vi "RIB Req - UDP Init.vi"(0 "Limits File Path":path, 5 "Results File Path":path, 11 "error in":errorcluster) -> (4 "Results Data Array":string[][](array[string]), 15 "error out":errorcluster)   [LabVIEW 2024]
doc: "Template test"
uses:
  <vilib>/addons/_JKI Toolkits/State Machine/_JKI_lib_State_Machine.llb/Select State(s)_err__jki_lib_state_machine.vi
  <vilib>/DAQmx/write.llb/DAQmx Write (Digital 1D Bool 1Chan 1Samp).vi
  <vilib>/addons/_JKI Toolkits/State Machine/_JKI_lib_State_Machine.llb/Select State(s)_bool__jki_lib_state_machine.vi
  <vilib>/DAQmx/read.llb/DAQmx Read (Digital 1D Bool 1Chan 1Samp).vi
  <vilib>/addons/_JKI Toolkits/State Machine/_JKI_lib_State_Machine.llb/Periodic Trigger__ogtk__JKI-SM__jki_lib_state_machine.vi
  <userlib>/_OpenG.lib/file/file.llb/Strip Path Extension - String__ogtk.vi
  <vilib>/Utility/file.llb/Read Delimited Spreadsheet (string).vi
  <vilib>/Utility/file.llb/Write Delimited Spreadsheet (string).vi
  <vilib>/DAQmx/create/channels.llb/DAQmx Create Channel (DO-Digital Output).vi
  <vilib>/DAQmx/miscellaneous.llb/DAQmx Fill In Error Info.vi
  <userlib>/_OpenG.lib/file/file.llb/openg_file.lvlib
  <userlib>/_OpenG.lib/appcontrol/appcontrol.llb/openg_application_control.lvlib
  <userlib>/_OpenG.lib/time/time.llb/openg_time.lvlib
panel:
  in  "Connect":string
  in  "Connect Fail":string
  out "data out":string
  out "Timeout (Read States) 4":dbl(slide) scale=0.0..10.0
  out "Timeout (Read States) 3":dbl(slide) scale=0.0..10.0
  out "Timeout (Read States) 2":dbl(slide) scale=0.0..10.0
  out "Timeout (Read States)":dbl(slide) scale=0.0..15.0
  out "element":string
  out "5A Test":bool
  out "ROV A Enabled":bool
  out "ROV B Enabled":bool
  out "TMS Enabled":bool
  out "Wait for Start":bool
  out "Normal Operation":bool
  in  "Read Normal Operation":string
  in  "Read Wait for Start":string
  in  "Read TMS":string
  in  "Read ROV B":string
  in  "Read ROV A":string
  out "Results Data 10":string[](array[string])
  out "Results Data 9":string[](array[string])
  out "Results Data 8":string[](array[string])
  out "Results Data 7":string[](array[string])
  out "Results Data 6":string[](array[string])
  out "Results Data 5":string[](array[string])
  out "Results Data 4":string[](array[string])
  in  "5A Test":bool
  out "Results Data 3":string[](array[string])
  in  "task out":refnum<k21>
  out "Timeout (5A)":dbl(slide) scale=0.0..5.0
  out "Timeout (Read UDP)":dbl(slide) scale=0.0..20.0
  out "Results Data 2":string[](array[string])
  in  "UDP Read":string
  in  "connection ID":refnum<k16>
  in  "Exit":bool
  # "UDP Initialise Test"
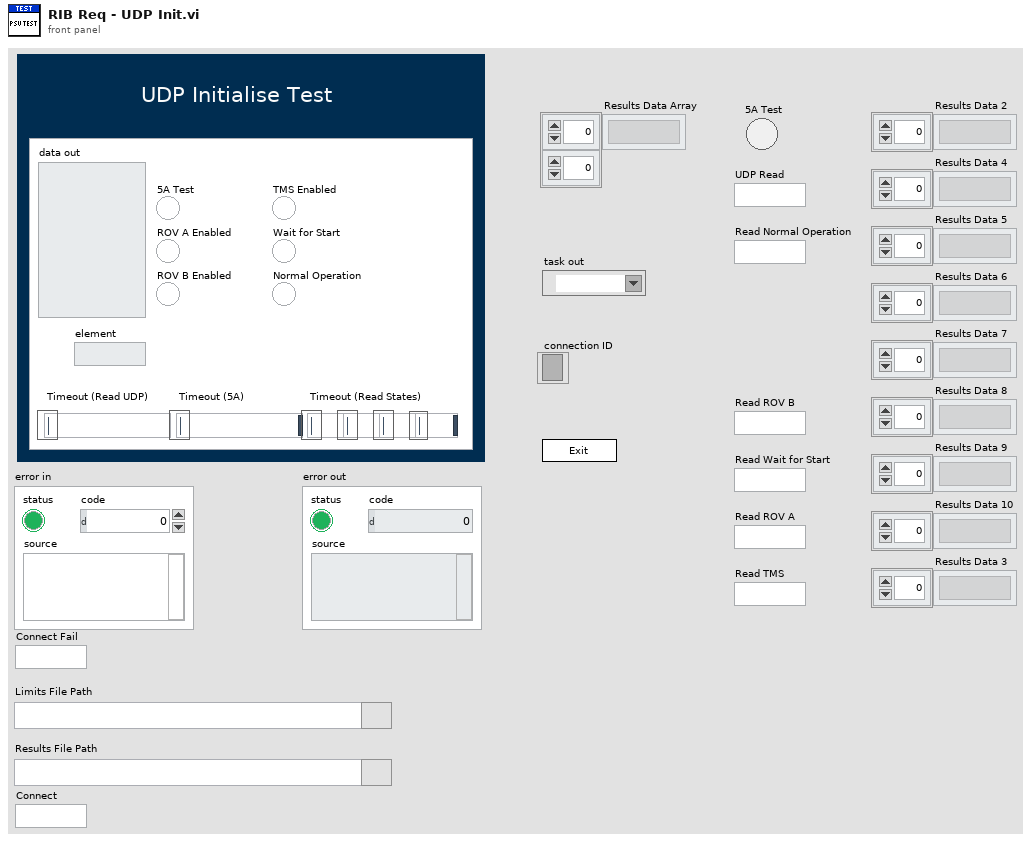
[diagram p1: front panel]
types:
  T1 = enum32{"Invalid", "Standard", "Closed", "Hidden", "Minimized", "Maximized"}
  T2 = enum32{"invalid app kind", "Development System", "Run Time System", "Student Edition", "Embedded LabVIEW", "Evaluation", "Custom"}
  T3 = typedef "FGV - Enum" = enum16{"Cleanup", "Get Data", "Open UDP", "Initialise DAQ", "Initialise I2C"}
  T4 = enum16{"Start Timer", "Get Time", "Pause", "Unpause"}
  T5 = cluster{"Core":cluster{"Current VI Reference":refnum<vi>, "Close Panel on Exit?":bool}, "Limits File Path":path, "Test Limits":string[][], "Results Data Array":string[][], "Results File Path":path, "UDP Read":string, "connection ID":refnum<k16>, "task out":refnum<k21>, "5A Test":bool, "Connect Fail":string, "Connect":string, "Read ROV A":string, "Read ROV B":string, "Read TMS":string, "Read Wait for Start":string, "Read Normal Operation":string}
  T6 = cluster{"Current VI Reference":refnum<vi>, "Close Panel on Exit?":bool}
  T7 = cluster{"[0]":bool, "[1]":bool, "[2]":bool, "[3]":bool, "[4]":bool, "[5]":bool, "[6]":bool, "[7]":bool, "[8]":bool}
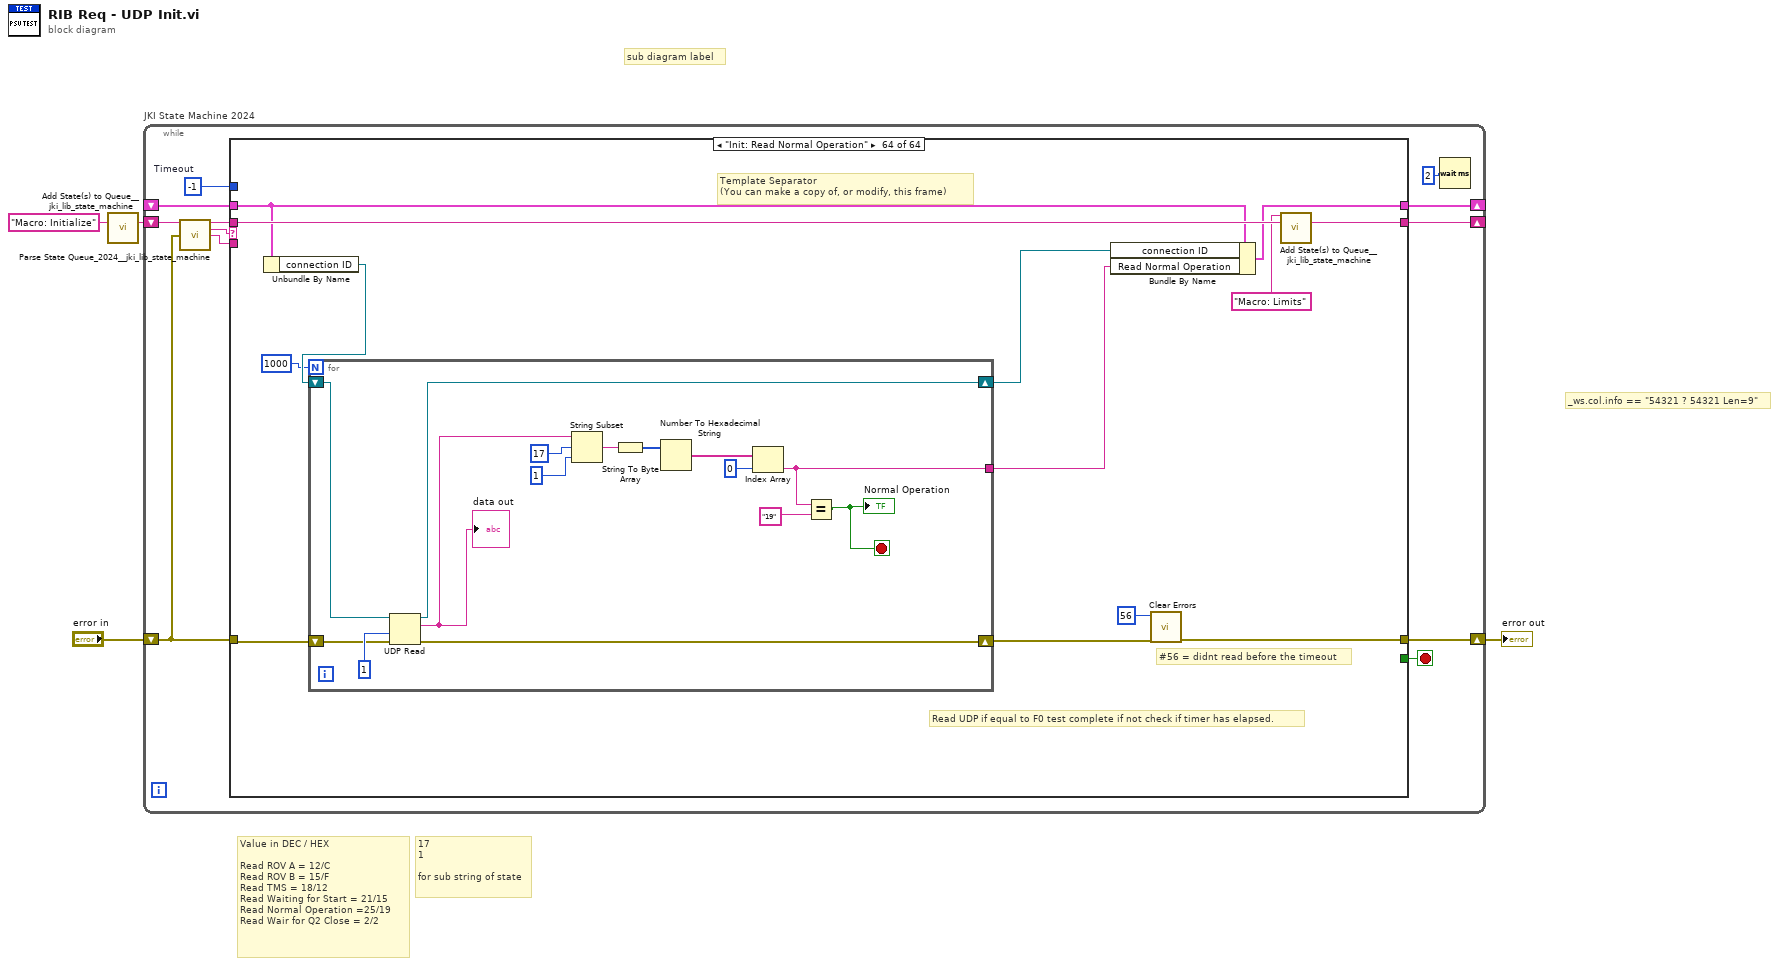
[diagram p0: block diagram]
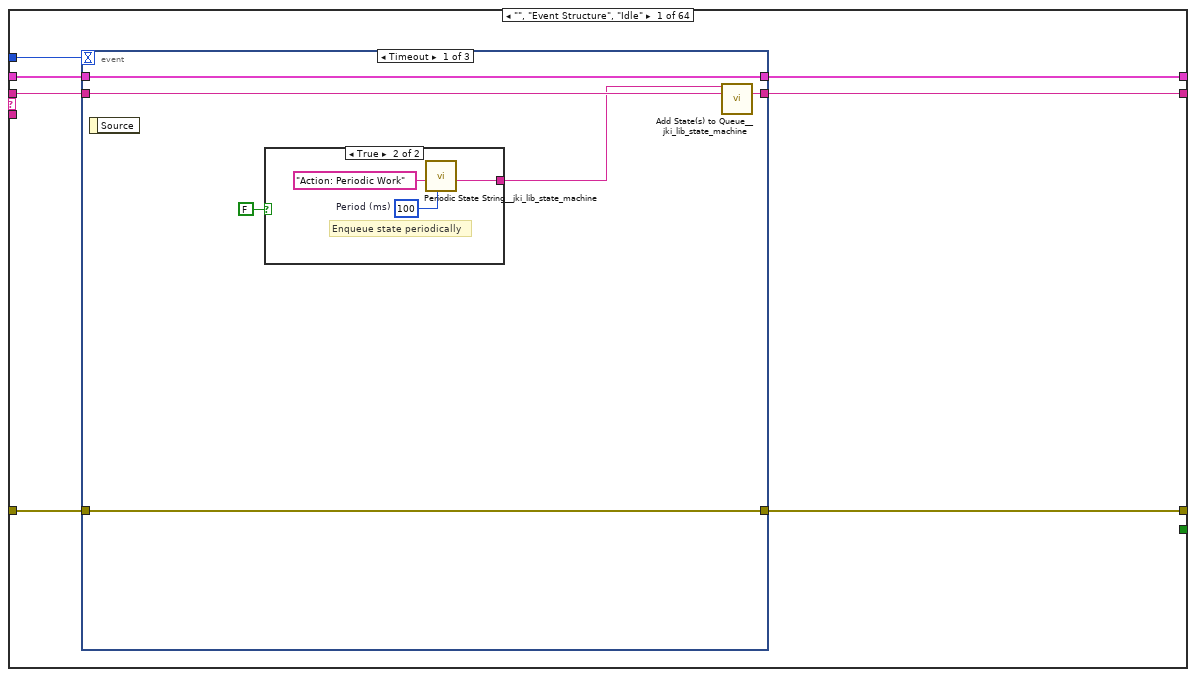
[diagram p2: hidden frame]
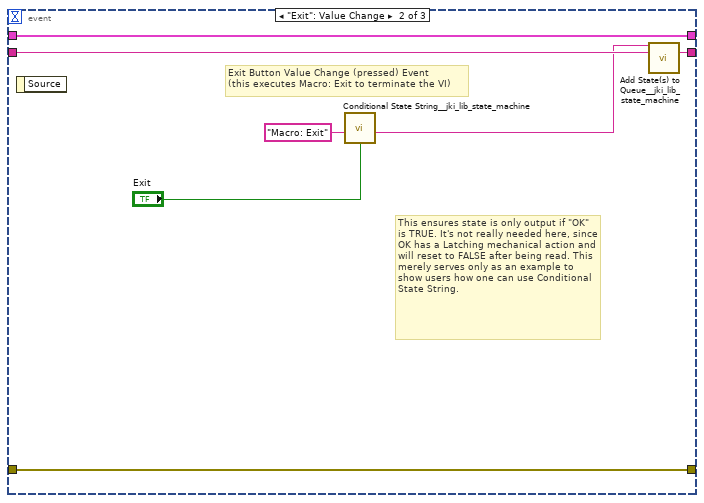
[diagram p4: hidden frame]
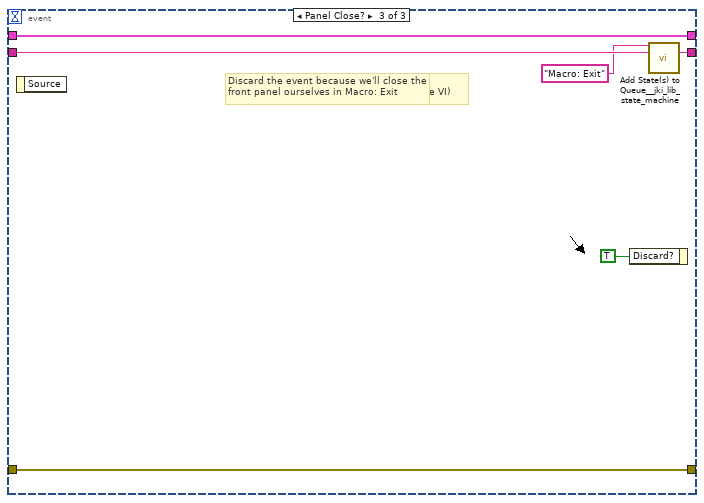
[diagram p5: hidden frame]
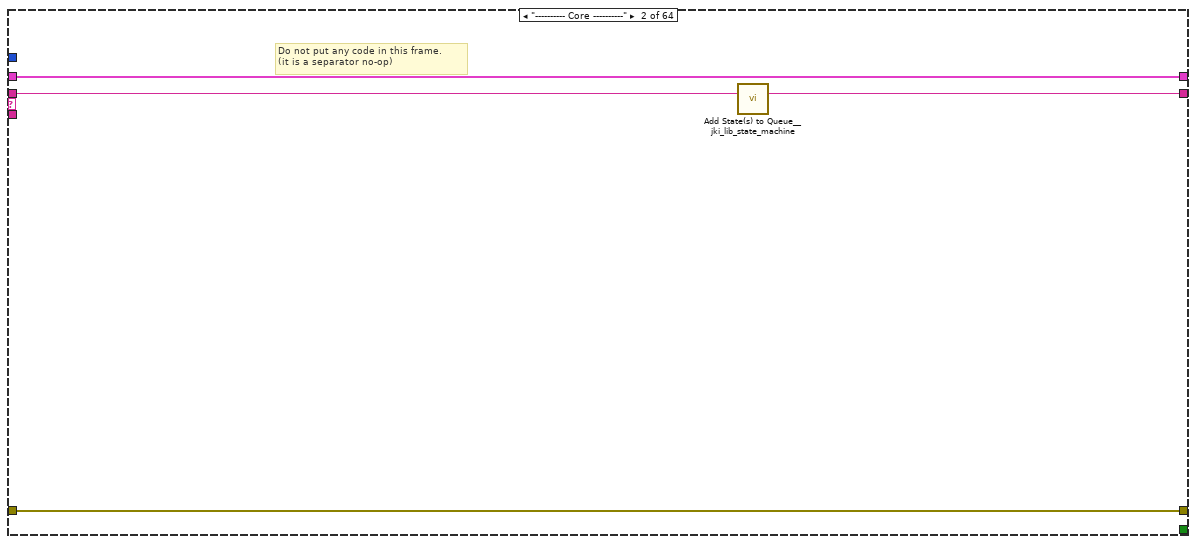
[diagram p6: hidden frame]
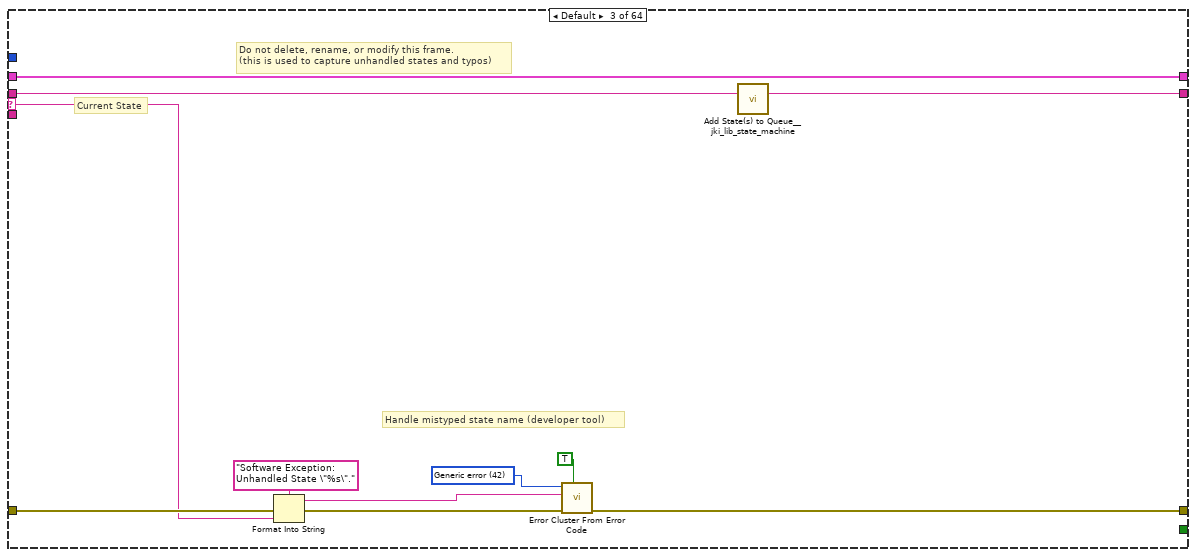
[diagram p7: hidden frame]
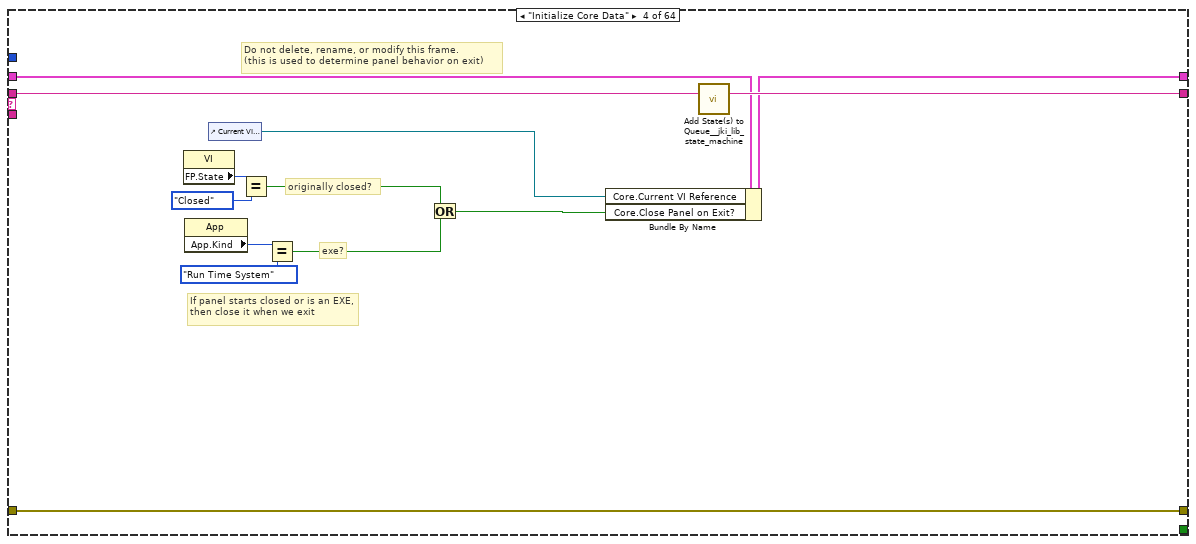
[diagram p8: hidden frame]
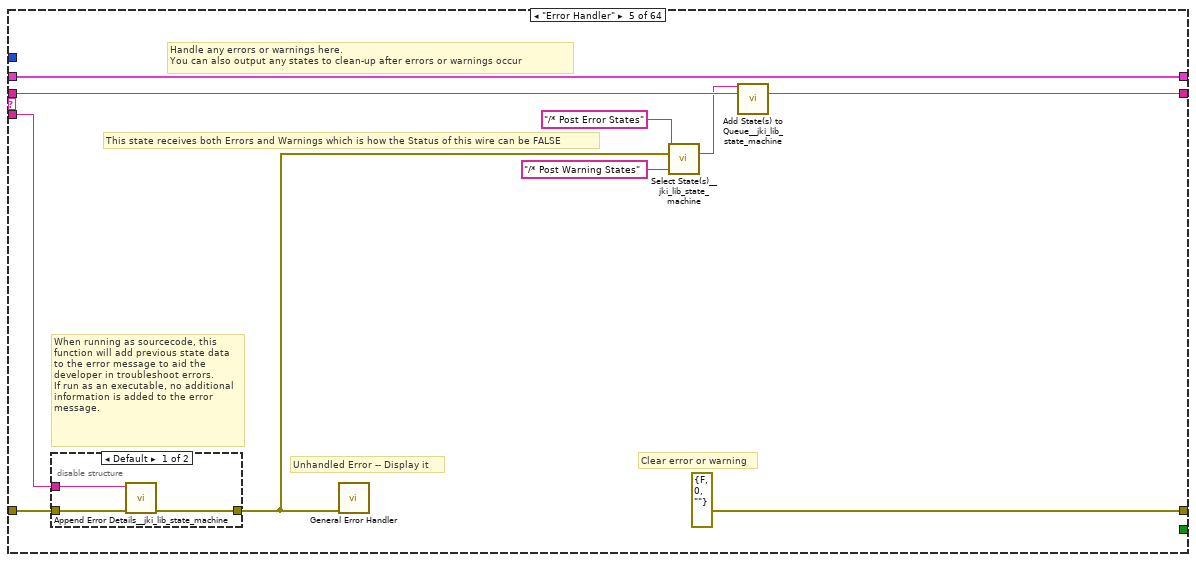
[diagram p9: hidden frame]
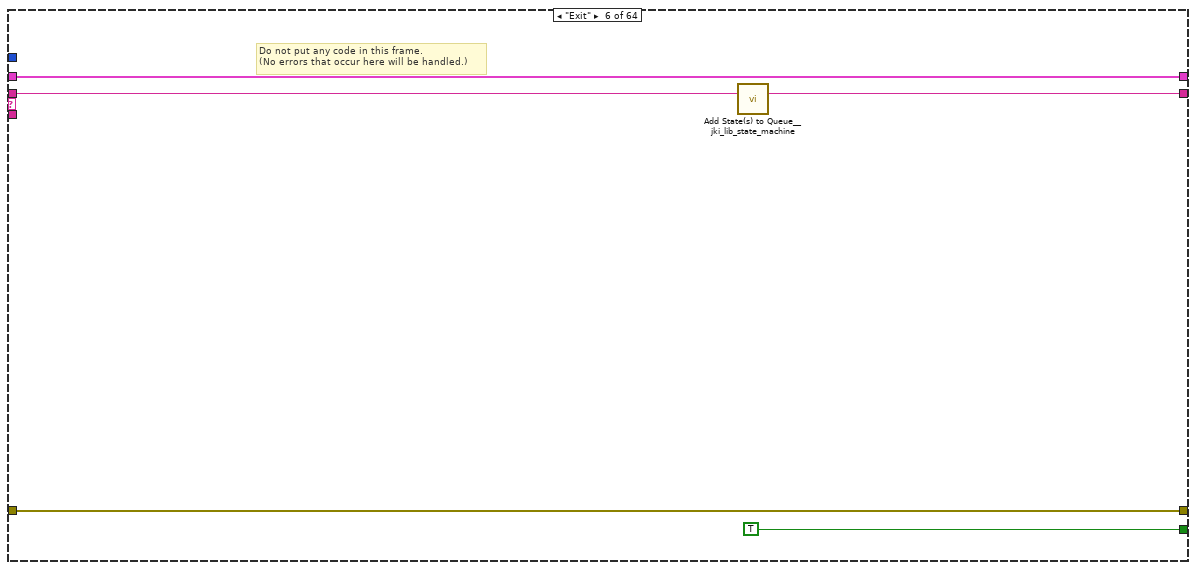
[diagram p11: hidden frame]
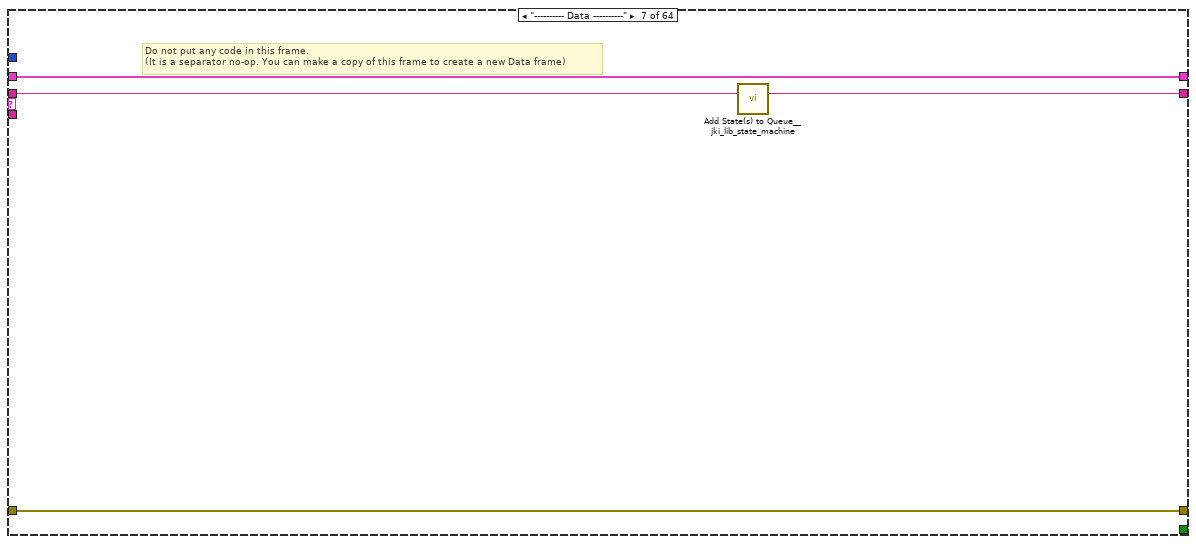
[diagram p12: hidden frame]
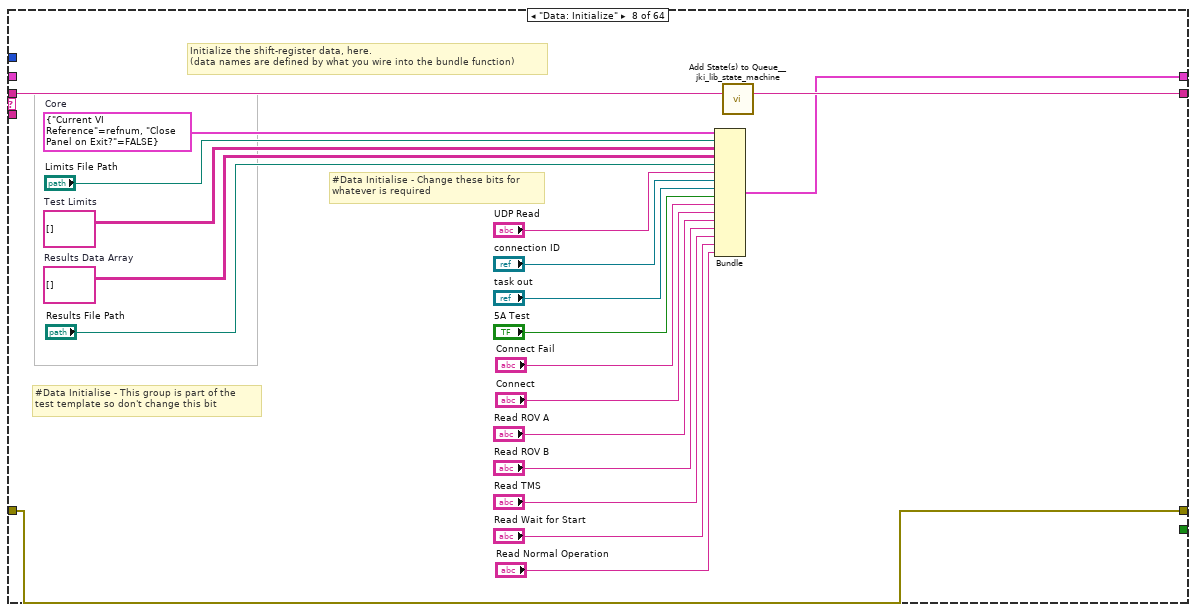
[diagram p13: hidden frame]
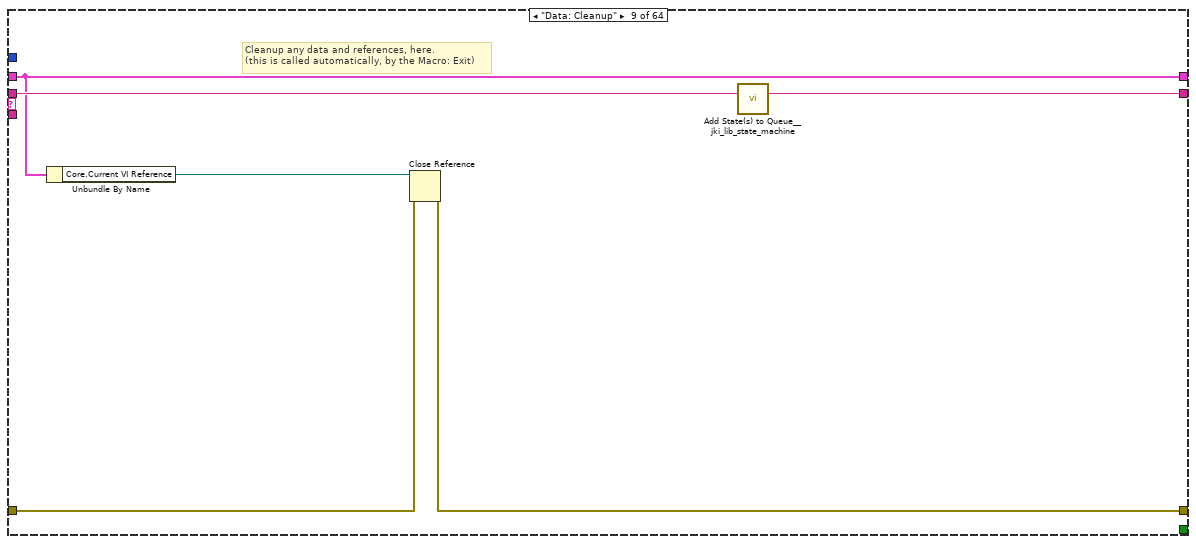
[diagram p14: hidden frame]
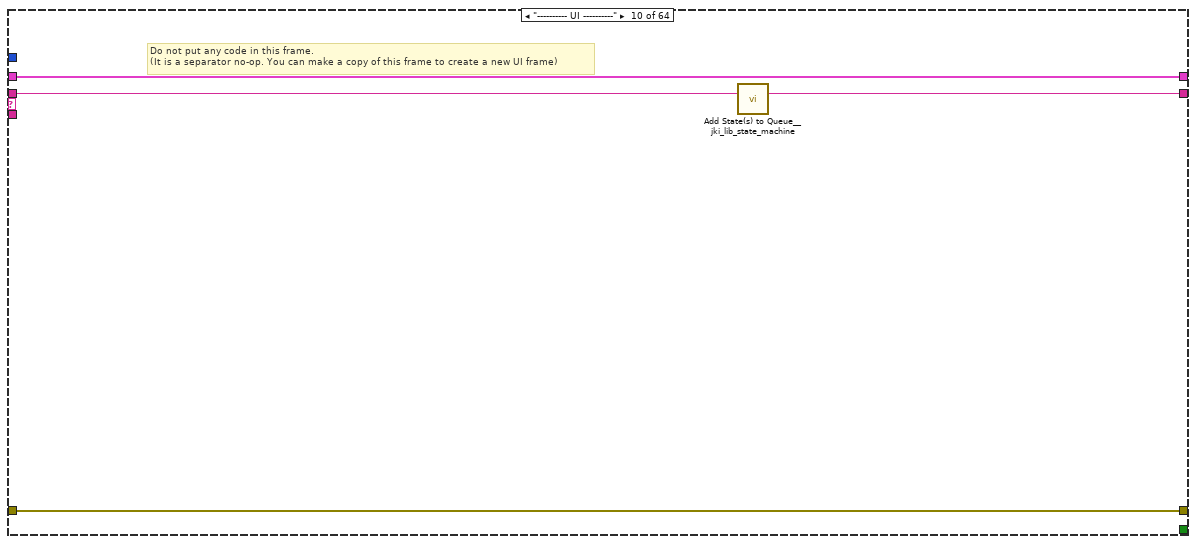
[diagram p15: hidden frame]
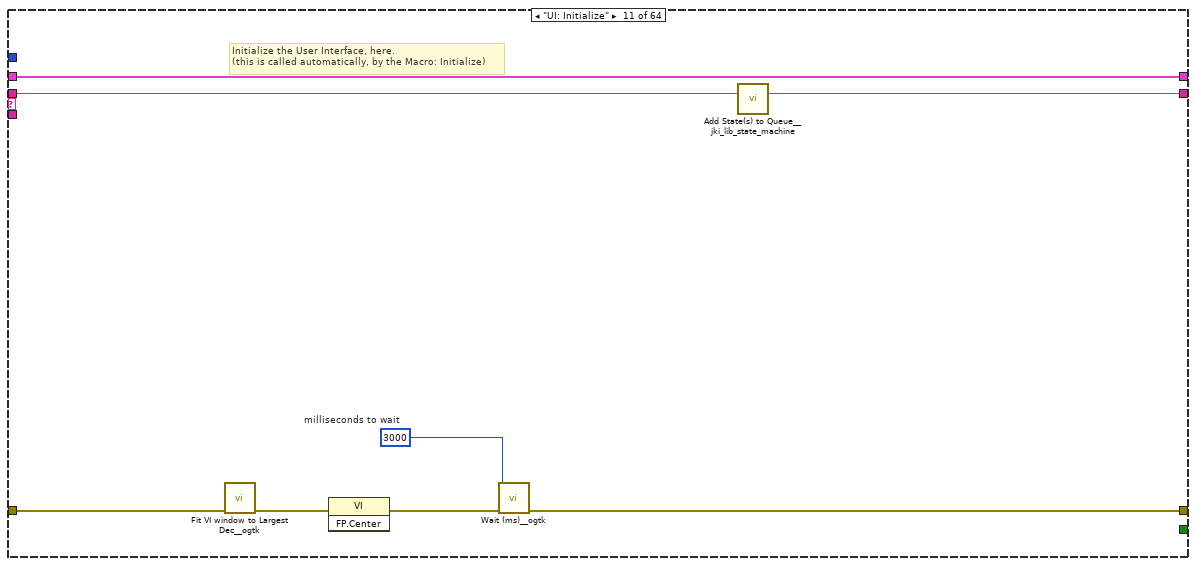
[diagram p16: hidden frame]
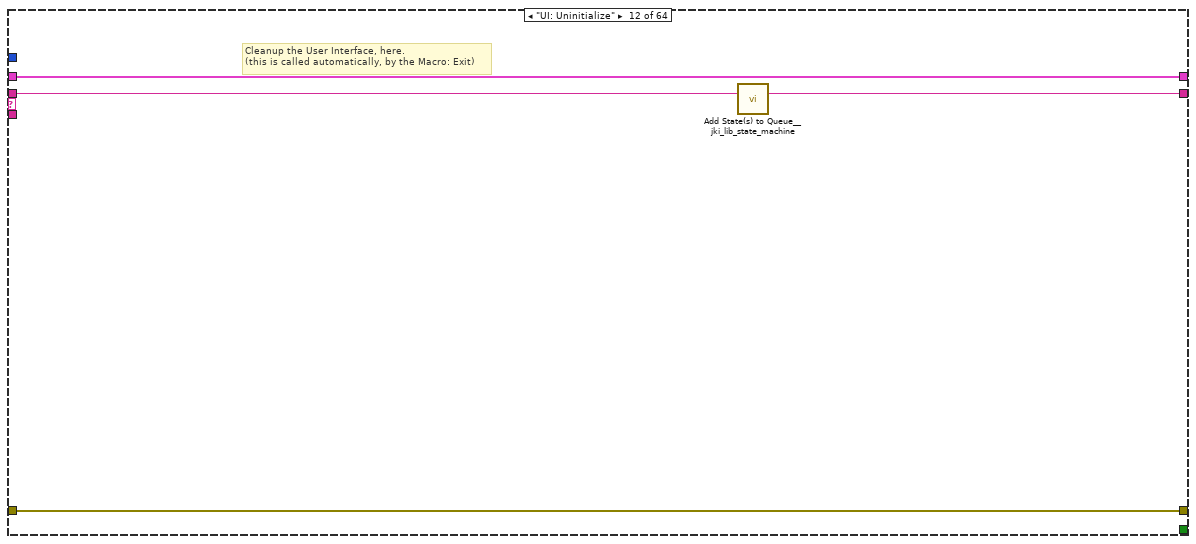
[diagram p17: hidden frame]
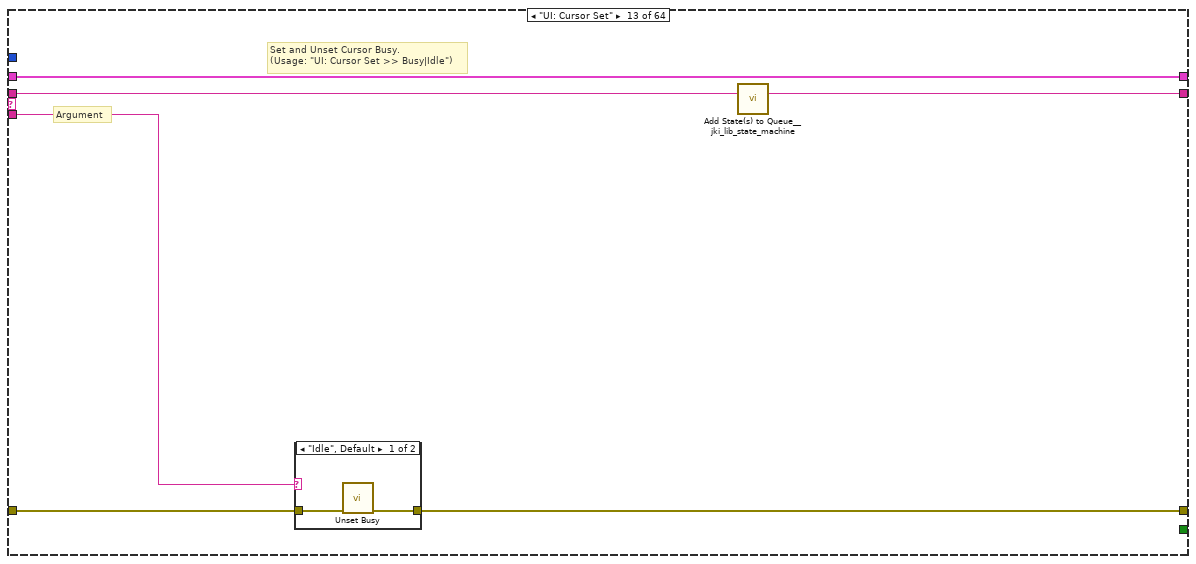
[diagram p18: hidden frame]
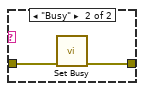
[diagram p19: hidden frame]
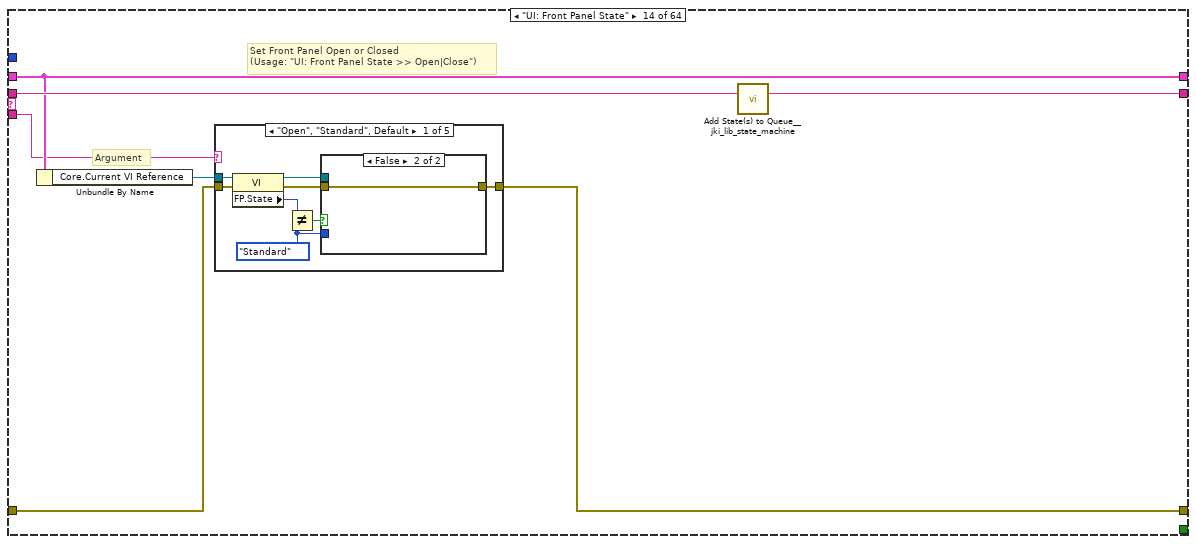
[diagram p20: hidden frame]
diagram:
  # "17\n1\n\nfor sub string of state"
  # "Value in DEC / HEX\n\nRead ROV A = 12/C\nRead ROV B = 15/F\nRead TMS = 18/12\nRead Waiting for Start = 21/15\nRead Normal Operation =25/19 \nRead Wair for Q2 Close = 2/2"
  # "_ws.col.info == \"54321 ? 54321 Len=9\""
  # "sub diagram label"
  n1 = call <vilib>:"Add State(s) to Queue__jki_lib_state_machine.vi"("State(s) in (\"\")"="Macro: Initialize") -> ("States Out"=w4:string)  [unwired: 14 in]
  n2 = while "JKI State Machine 2024" {
    shift-right: [w9] -> _
    shift-left: _ -> [w8]
    shift-right: [w12] -> w1
    shift-left: "error in" -> [w6]
    shift-right: [w11] -> _
    shift-left: w4 -> [w13]
    stop <- w10 stop-if-true
    w7 = -1  # Timeout
    n3 = call <vilib>:"Parse State Queue_2024__jki_lib_state_machine.vi"("State Queue"=w13, "Error In (no error)"=w6) -> ("Remaining States"=w15:string, "Current State"=w16:string, "Arguments"=w14:string)  [unwired: 11 in]
    n4 = case shown="\"Init: Read Normal Operation\"" w16 {
      selector: w16 -> [_ _ w50 _ _ _ _ _ _ _ _ _ _ _ _ _ _ _ _ _ _ _ _ _ _ _ _ _ _ _ _ _ _ _ _ _ _ _ _ _ _ _ _ _ _ _ _ _ _ _ _ _ _ _ _ _ _ _ _ _ _ _ _ _]
      tunnel: w15 -> [w23 w49 w54 w73 w83 w92 w96 w116 w122 w126 w134 w138 w144 w155 w224 w229 w234 w239 w248 w252 w265 w282 w295 w308 w321 w334 w347 w360 w373 w386 w390 w399 w403 w419 w426 w439 w448 w473 w499 w524 w550 w561 w582 w606 w618 w629 w649 w661 w706 w728 w739 w763 w775 w786 w810 w822 w833 w857 w869 w880 w904 w916 w938 w951]
      tunnel: w14 -> [_ _ _ _ w78 _ _ _ _ _ _ _ w139 w149 _ _ _ _ _ _ _ _ _ _ _ _ _ _ _ _ _ _ _ _ _ _ _ _ _ _ _ _ _ _ _ _ _ _ _ _ _ _ _ _ _ _ _ _ _ _ _ _ _ _]
      tunnel: w8 -> [w21 w46 w52 w66 w80 w90 w93 _ w117 w123 w132 w136 w142 w151 w221 w226 w231 w236 w246 w249 w255 w274 w287 w300 w313 w326 w339 w352 w365 w378 w387 w395 w400 w417 w422 w434 w446 w454 w495 w505 w546 w559 w565 w600 w616 w627 w645 w659 w670 w725 w737 w749 w773 w784 w793 w820 w831 w840 w867 w878 w887 w914 w935 w946]
      tunnel: [w20 w47 w56 w70 errorcluster {"status"=FALSE, "code"=0, "source"=""} ("error out") w89 w94 w113 w118 w124 w130 w135 w140 w152 w222 w227 w232 w237 w243 w250 w261 w279 w292 w305 w318 w331 w344 w357 w370 w383 w388 w397 w401 w407 w421 w430 w443 w450 w490 w501 w542 w552 w562 w586 w613 w619 w634 w656 w664 w708 w730 w747 w770 w777 w789 w817 w824 w836 w864 w871 w883 w911 w918 w943] -> w12
      tunnel: w6 -> [w17 w47 w55 w70 w79 w89 w94 w113 w119 w124 w131 w135 w141 w153 w222 w227 w232 w237 w243 w250 w260 w278 w291 w304 w317 w330 w343 w356 w369 w382 w388 w396 w401 w412 w421 w435 w442 w455 w497 w506 w548 w557 w567 w602 w614 w625 w635 w657 w673 w714 w735 w746 w771 w782 w788 w818 w829 w835 w865 w876 w882 w912 w924 w945]
      tunnel: [w22 w48 w53 w72 w82 w91 w95 w115 w121 w125 w133 w137 w143 w154 w223 w228 w233 w238 w247 w251 w264 w281 w294 w307 w320 w333 w346 w359 w372 w385 w389 w398 w402 w418 w425 w438 w447 w472 w498 w523 w549 w560 w581 w605 w617 w628 w648 w660 w705 w727 w738 w762 w774 w785 w809 w821 w832 w856 w868 w879 w903 w915 w937 w950] -> w11
      tunnel: [_ _ _ _ _ TRUE _ _ _ _ _ _ _ _ _ _ _ _ _ _ _ _ _ _ _ _ _ _ _ _ _ _ _ _ _ _ _ _ _ _ _ _ _ _ _ _ _ _ _ _ _ _ _ _ _ _ _ _ _ _ _ _ _ _] -> w10
      tunnel: [w19 w46 w52 w71 w80 w90 w93 w114 w117 w123 w132 w136 w142 w151 w221 w226 w231 w236 w246 w249 w254 w273 w286 w299 w312 w325 w338 w351 w364 w377 w387 w395 w400 w417 w422 w433 w445 w456 w494 w507 w545 w559 w569 w599 w616 w627 w644 w659 w704 w726 w737 w748 w773 w784 w792 w820 w831 w839 w867 w878 w886 w914 w936 w941] -> w9
      tunnel: w7 -> [w18 _ _ _ _ _ _ _ _ _ _ _ _ _ _ _ _ _ _ _ _ _ _ _ _ _ _ _ _ _ _ _ _ _ _ _ _ _ _ _ _ _ _ _ _ _ _ _ _ _ _ _ _ _ _ _ _ _ _ _ _ _ _ _]
      frame "", "Event Structure", "Idle" {
        n5 = event shown="[0] Timeout" {
          selector: _ -> [_ _ _]
          dyn-events: _ -> [_ _ _]
          timeout: w18 -> [_ _ _]
          tunnel: w23 -> [w29 w39 w45]
          tunnel: [w28 w38 w44] -> w22
          tunnel: w21 -> [w26 w36 w42]
          tunnel: [w27 w37 w43] -> w20
          tunnel: w17 -> [w27 w37 w43]
          tunnel: [w26 w36 w42] -> w19
          event Timeout {
            n6 = event-data() -> ()  [unwired: 1 in, 1 out]
            n7 = case shown="True" FALSE {
              tunnel: [_ w32] -> w25
              frame False {
              }
              frame True {
                w30 = u32 100  # Period (ms)
                # "Enqueue state periodically"
                n8 = call <vilib>:"Periodic State String__jki_lib_state_machine.vi"("Period (ms)"=w30, "State"="Action: Periodic Work") -> ("State Out"=w32:string)  [unwired: 9 in]
              }
            }
            n9 = call <vilib>:"Add State(s) to Queue__jki_lib_state_machine.vi"("State(s) in Front (\"\")"=w25, "State(s) in (\"\")"=w29) -> ("States Out"=w28:string)  [unwired: 13 in]
          }
          event "Exit": Value Change {
            # "This ensures state is only output if \"OK\" is TRUE. It's not really needed here, since OK has a Latching mechanical action and will reset to FALSE after being read. This merely serves only as an example to show users how one can use Conditional State String."
            # "Exit Button Value Change (pressed) Event\n(this executes Macro: Exit to terminate the VI)"
            n10 = event-data() -> ()  [unwired: 1 in, 1 out]
            n11 = call <vilib>:"Conditional State String__jki_lib_state_machine.vi"("Do State(s)?"="Exit", "State"="Macro: Exit") -> ("State Out"=w33:string)  [unwired: 7 in]
            n12 = call <vilib>:"Add State(s) to Queue__jki_lib_state_machine.vi"("State(s) in Front (\"\")"=w33, "State(s) in (\"\")"=w39) -> ("States Out"=w38:string)  [unwired: 13 in]
          }
          event Panel Close? {
            # "Discard the event because we'll close the front panel ourselves in Macro: Exit"
            # "Close Panel button (pressed) Event\n(this executes Macro: Exit to terminate the VI)"
            n13 = event-data() -> ()  [unwired: 1 in, 1 out]
            n14 = event-data("Discard?"=TRUE) -> ()  [unwired: 1 in, 1 out]
            n15 = call <vilib>:"Add State(s) to Queue__jki_lib_state_machine.vi"("State(s) in Front (\"\")"="Macro: Exit", "State(s) in (\"\")"=w45) -> ("States Out"=w44:string)  [unwired: 13 in]
          }
        }
      }
      frame "---------- Core ----------" {
        # "Do not put any code in this frame.\n(it is a separator no-op)"
        n16 = call <vilib>:"Add State(s) to Queue__jki_lib_state_machine.vi"("State(s) in (\"\")"=w49) -> ("States Out"=w48:string)  [unwired: 14 in]
      }
      frame Default {
        w59 = 42 items=["No error", "Argument error", "Memory is full", "Out of zone", "End of file", "File already open", "Generic file I/O error", "File not found", "File permission error", "Disk is full", "Duplicate path", "Too many files open", "System feature not enabled", "Resource file not found", "Cannot add resource", "Resource not found", "Image not found", "Image memory error", "Pen does not exist", "Config type invalid", "Config token not found", "Config parse error", "Config memory error", "Bad external code format", "Bad external code offset", "External code not present", "Null window", "Destroy window error", "Null menu", "Print aborted", "Bad print record", "Print driver error", "Windows error during printing", "Memory error during printing", "Print dialog error", "Generic print error", "Invalid device refnum", "Device not found", "Device parameter error", "Device unit error", "Cannot open device", "Device call aborted", "Generic error", "Cancelled by user", "Object ID too low", "Object ID too high", "Object not in heap", "Unknown heap", "Unknown object (invalid DefProc)", "Unknown object (DefProc not in table)", "Message out of range", "Invalid (null) method", "Unknown message", "Manager call not supported", "Bad address", "Network operation in progress", "Network operation timed out", "Connection is busy", "Network attribute not supported", "Network error", "Address in use", "System out of memory", "Connection aborted", "Connection refused", "Not connected", "Already connected", "Connection closed", "Initialization error (interapplication manager)", "Bad occurrence", "Wait on unbound occurrence handler", "Occurrence queue overflow", "Datalog type conflict", "Unused", "Unrecognized type (interapplication manager)", "Memory corrupt", "Failed to make temporary DLL", "Old CIN version", "Drag socket not found", "Failed to load drop-object", "Failed to register OLE object", "Failed to release OLE object", "Format specifier type mismatch", "Unknown format specifier", "Too few format specifiers", "Too many format specifiers", "Scan failed", "Newer CIN version", "Error converting to variant", "Runtime menu error", "Password tampered", "Variant attribute not found", "Incompatible variant data type", "Event data is not available", "Event Store is not present", "Occurrence is not found", "Event Queue is not created", "Event info is not available", "Refnum passed is NULL", "Error retrieving Class GUID", "Error retrieving CoClass GUID", "Error retrieving TypeLib GUID.", "Bad built application magic bytes.", "Specific driver is different from the specific driver associated with the Logical Name.", "There is no session opened to the class driver.", "Max Error", "MAX - Error with config objects", "MAX - Error loading configuration", "MAX - Group not supported"]
        # "Current State"
        # "Do not delete, rename, or modify this frame.\n(this is used to capture unhandled states and typos)"
        # "Handle mistyped state name (developer tool)"
        n17 = Format Into String(format string="Software Exception: Unhandled State \"%s\"." ("message"), error in=w55, w50) -> (resulting string=w58:string, error out=w57:errorcluster)  [unwired: 1 in]
        n18 = call <vilib>:"Error Cluster From Error Code.vi"("show call chain? (False)"=TRUE, "error in (no error)"=w57, "error message (\"\")"=w58, "error code (0)"=w59) -> ("error out"=w56:errorcluster)  [unwired: 5 in]
        n19 = call <vilib>:"Add State(s) to Queue__jki_lib_state_machine.vi"("State(s) in (\"\")"=w54) -> ("States Out"=w53:string)  [unwired: 14 in]
      }
      frame "Initialize Core Data" {
        # "Do not delete, rename, or modify this frame.\n(this is used to determine panel behavior on exit)"
        # "originally closed?"
        # "exe?"
        # "If panel starts closed or is an EXE, then close it when we exit"
        n20 = property class="VI"() -> ("FP.State"=w63:T1)  [unwired: 2 in, 2 out]
        n21 = property class="App"() -> ("App.Kind"=w69:T2)  [unwired: 2 in, 2 out]
        n22 = control-ref of="Current VI Reference"() -> (w64:refnum<vi>)
        n23 = Equal?(x=w63, y=T1."Closed" ("Front Panel Window:State")) -> (x = y?=w61:bool)
        n24 = Equal?(x=w69, y=T2."Run Time System" ("Application:Kind")) -> (x = y?=w67:bool)
        n25 = Or(x=w61, y=w67) -> (x .or. y?=w65:bool)
        n26 = Bundle By Name(cluster=w66, "Core.Current VI Reference"=w64, "Core.Close Panel on Exit?"=w65) -> (w71:T5)
        n27 = call <vilib>:"Add State(s) to Queue__jki_lib_state_machine.vi"("State(s) in (\"\")"=w73) -> ("States Out"=w72:string)  [unwired: 14 in]
      }
      frame "Error Handler" {
        # "When running as sourcecode, this function will add previous state data to the error message to aid the developer in troubleshoot errors.\nIf run as an executable, no additional information is added to the error message."
        # "This state receives both Errors and Warnings which is how the Status of this wire can be FALSE"
        # "Unhandled Error -- Display it"
        # "Handle any errors or warnings here.\nYou can also output any states to clean-up after errors or warnings occur"
        # "Clear error or warning"
        n28 = disable-structure shown="Default" {
          disable-tunnel: w79 -> [w86 w87]
          disable-tunnel: w78 -> [w85 _]
          disable-tunnel: [w84 w87] -> w77
          frame condition #0 (active) {
            n29 = call <vilib>:"Append Error Details__jki_lib_state_machine.vi"("error in (no error)"=w86, "Previous State and Argument(s)"=w85) -> ("error out"=w84:errorcluster)  [unwired: 9 in]
          }
          frame condition #1 {
          }
        }
        n30 = call <vilib>:"General Error Handler.vi"("error in (no error)"=w77) -> ()  [unwired: 10 in, 5 out]
        n31 = call-poly <vilib>:"Select State(s)__jki_lib_state_machine.vi"("State(s) if True (\"\")"="/* Post Error States", "Select"=w77, "State(s) if False (\"\")"="/* Post Warning States") -> ("States Out"=w75:string)  [unwired: 12 in]
        n32 = call <vilib>:"Add State(s) to Queue__jki_lib_state_machine.vi"("State(s) in Front (\"\")"=w75, "State(s) in (\"\")"=w83) -> ("States Out"=w82:string)  [unwired: 13 in]
      }
      frame "Exit" {
        # "Do not put any code in this frame.\n(No errors that occur here will be handled.)"
        n33 = call <vilib>:"Add State(s) to Queue__jki_lib_state_machine.vi"("State(s) in (\"\")"=w92) -> ("States Out"=w91:string)  [unwired: 14 in]
      }
      frame "---------- Data ----------" {
        # "Do not put any code in this frame.\n(It is a separator no-op. You can make a copy of this frame to create a new Data frame)"
        n34 = call <vilib>:"Add State(s) to Queue__jki_lib_state_machine.vi"("State(s) in (\"\")"=w96) -> ("States Out"=w95:string)  [unwired: 14 in]
      }
      frame "Data: Initialize" {
        w109 = string[][] []  # Results Data Array
        w110 = string[][] []  # Test Limits
        w112 = T6 {"Current VI Reference"=refnum, "Close Panel on Exit?"=FALSE}  # Core
        # "#Data Initialise - Change these bits for\nwhatever is required"
        # "#Data Initialise - This group is part of the\ntest template so don't change this bit"
        # "Initialize the shift-register data, here.\n(data names are defined by what you wire into the bundle function)"
        n35 = Bundle("Core"=w112, "Limits File Path"="Limits File Path", "Test Limits"=w110, "Results Data Array"=w109, "Results File Path"="Results File Path", "UDP Read"="UDP Read", "connection ID"="connection ID", "task out"="task out", "5A Test"="5A Test", "Connect Fail"="Connect Fail", "Connect"="Connect", "Read ROV A"="Read ROV A", "Read ROV B"="Read ROV B", "Read TMS"="Read TMS", "Read Wait for Start"="Read Wait for Start", "Read Normal Operation"="Read Normal Operation") -> (w114:T5)  [unwired: 1 in]
        n36 = call <vilib>:"Add State(s) to Queue__jki_lib_state_machine.vi"("State(s) in (\"\")"=w116) -> ("States Out"=w115:string)  [unwired: 14 in]
      }
      frame "Data: Cleanup" {
        # "Cleanup any data and references, here.\n(this is called automatically, by the Macro: Exit)"
        n37 = Unbundle By Name(w117) -> ("Core.Current VI Reference"=w120:refnum<vi>)
        n38 = Close Reference(reference=w120, error in (no error)=w119) -> (error out=w118:errorcluster)
        n39 = call <vilib>:"Add State(s) to Queue__jki_lib_state_machine.vi"("State(s) in (\"\")"=w122) -> ("States Out"=w121:string)  [unwired: 14 in]
      }
      frame "---------- UI ----------" {
        # "Do not put any code in this frame.\n(It is a separator no-op. You can make a copy of this frame to create a new UI frame)"
        n40 = call <vilib>:"Add State(s) to Queue__jki_lib_state_machine.vi"("State(s) in (\"\")"=w126) -> ("States Out"=w125:string)  [unwired: 14 in]
      }
      frame "UI: Initialize" {
        w129 = u32 3000  # milliseconds to wait
        # "Initialize the User Interface, here.\n(this is called automatically, by the Macro: Initialize)"
        n41 = call <userlib>:"Fit VI window to Largest Dec__ogtk.vi"("error in (no error)"=w131) -> ("error out"=w127:errorcluster)  [unwired: 5 in, 1 out]
        n42 = invoke class="VI" method="FP.Center"(error in=w127) -> (error out=w128:errorcluster)  [unwired: 2 in, 2 out]
        n43 = call <userlib>:"Wait (ms)__ogtk.vi"("error in (no error)"=w128, "milliseconds to wait"=w129) -> ("error out"=w130:errorcluster)  [unwired: 8 in, 1 out]
        n44 = call <vilib>:"Add State(s) to Queue__jki_lib_state_machine.vi"("State(s) in (\"\")"=w134) -> ("States Out"=w133:string)  [unwired: 14 in]
      }
      frame "UI: Uninitialize" {
        # "Cleanup the User Interface, here.\n(this is called automatically, by the Macro: Exit)"
        n45 = call <vilib>:"Add State(s) to Queue__jki_lib_state_machine.vi"("State(s) in (\"\")"=w138) -> ("States Out"=w137:string)  [unwired: 14 in]
      }
      frame "UI: Cursor Set" {
        # "Argument"
        # "Set and Unset Cursor Busy.\n(Usage: \"UI: Cursor Set >> Busy|Idle\")"
        n46 = case shown="\"Idle\", Default" w139 {
          tunnel: w141 -> [w146 w148]
          tunnel: [w145 w147] -> w140
          frame "Idle", Default {
            n47 = call <vilib>:"Unset Busy.vi"("error in (no error)"=w146) -> ("error out"=w145:errorcluster)  [unwired: 10 in]
          }
          frame "Busy" {
            n48 = call <vilib>:"Set Busy.vi"("error in (no error)"=w148) -> ("error out"=w147:errorcluster)  [unwired: 9 in, 1 out]
          }
        }
        n49 = call <vilib>:"Add State(s) to Queue__jki_lib_state_machine.vi"("State(s) in (\"\")"=w144) -> ("States Out"=w143:string)  [unwired: 14 in]
      }
      frame "UI: Front Panel State" {
        # "Argument"
        # "Set Front Panel Open or Closed\n(Usage: \"UI: Front Panel State >> Open|Close\")"
        n50 = Unbundle By Name(w151) -> ("Core.Current VI Reference"=w150:refnum<vi>)
        n51 = case shown="\"Open\", \"Standard\", Default" w149 {
          tunnel: w153 -> [w161 w176 w187 w200 w213]
          tunnel: [w163 w177 w189 w202 w215] -> w152
          tunnel: w150 -> [w162 w174 w188 w201 w214]
          frame "Open", "Standard", Default {
            w156 = T1."Standard" ("State")
            n52 = property class="VI"(reference=w162, error in=w161) -> (reference out=w159:refnum<vi>, error out=w160:errorcluster, "FP.State"=w158:T1)
            n53 = Not Equal?(x=w158, y=w156) -> (x != y?=w157:bool)
            n54 = case shown="False" w157 {
              tunnel: [w167 w169] -> w163
              tunnel: w160 -> [w166 w169]
              tunnel: w159 -> [w165 _]
              tunnel: w156 -> [w164 _]
              frame True {
                n55 = invoke class="VI" method="FP.Open"(reference=w165, error in=w166, "Activate"=TRUE, "State"=w164) -> (error out=w167:errorcluster)  [unwired: 1 in, 4 out]
              }
              frame False {
              }
            }
          }
          frame "Close", "Closed" {
            n56 = property class="VI"(reference=w174, error in=w176) -> (reference out=w173:refnum<vi>, error out=w175:errorcluster, "FP.State"=w171:T1)
            n57 = Not Equal?(x=w171, y=T1."Closed" ("Front Panel Window:State")) -> (x != y?=w170:bool)
            n58 = case shown="True" w170 {
              tunnel: [w178 w181] -> w177
              tunnel: w175 -> [w178 w180]
              tunnel: w173 -> [_ w179]
              frame False {
              }
              frame True {
                n59 = invoke class="VI" method="FP.Close"(reference=w179, error in=w180) -> (error out=w181:errorcluster)  [unwired: 1 in, 2 out]
              }
            }
          }
          frame "Hidden", "Hide" {
            w182 = T1."Hidden" ("State")
            n60 = property class="VI"(reference=w188, error in=w187) -> (reference out=w185:refnum<vi>, error out=w186:errorcluster, "FP.State"=w184:T1)
            n61 = Not Equal?(x=w184, y=w182) -> (x != y?=w183:bool)
            n62 = case shown="True" w183 {
              tunnel: [w193 w194] -> w189
              tunnel: w186 -> [w192 w194]
              tunnel: w185 -> [w191 _]
              tunnel: w182 -> [w190 _]
              frame True {
                n63 = invoke class="VI" method="FP.Open"(reference=w191, error in=w192, "State"=w190) -> (error out=w193:errorcluster)  [unwired: 2 in, 4 out]
              }
              frame False {
              }
            }
          }
          frame "Minimize", "Minimized" {
            w195 = T1."Minimized" ("State")
            n64 = property class="VI"(reference=w201, error in=w200) -> (reference out=w198:refnum<vi>, error out=w199:errorcluster, "FP.State"=w197:T1)
            n65 = Not Equal?(x=w197, y=w195) -> (x != y?=w196:bool)
            n66 = case shown="True" w196 {
              tunnel: [w206 w207] -> w202
              tunnel: w199 -> [w205 w207]
              tunnel: w198 -> [w204 _]
              tunnel: w195 -> [w203 _]
              frame True {
                n67 = invoke class="VI" method="FP.Open"(reference=w204, error in=w205, "State"=w203) -> (error out=w206:errorcluster)  [unwired: 2 in, 4 out]
              }
              frame False {
              }
            }
          }
          frame "Maximize", "Maximized" {
            w208 = T1."Maximized" ("State")
            n68 = property class="VI"(reference=w214, error in=w213) -> (reference out=w211:refnum<vi>, error out=w212:errorcluster, "FP.State"=w210:T1)
            n69 = Not Equal?(x=w210, y=w208) -> (x != y?=w209:bool)
            n70 = case shown="True" w209 {
              tunnel: [w219 w220] -> w215
              tunnel: w212 -> [w218 w220]
              tunnel: w211 -> [w217 _]
              tunnel: w208 -> [w216 _]
              frame True {
                n71 = invoke class="VI" method="FP.Open"(reference=w217, error in=w218, "State"=w216) -> (error out=w219:errorcluster)  [unwired: 2 in, 4 out]
              }
              frame False {
              }
            }
          }
        }
        n72 = call <vilib>:"Add State(s) to Queue__jki_lib_state_machine.vi"("State(s) in (\"\")"=w155) -> ("States Out"=w154:string)  [unwired: 14 in]
      }
      frame "---------- Macro ----------" {
        # "Do not put any code in this frame.\n(It is a separator no-op. You can make a copy of this frame to create a new Macro frame)"
        n73 = call <vilib>:"Add State(s) to Queue__jki_lib_state_machine.vi"("State(s) in (\"\")"=w224) -> ("States Out"=w223:string)  [unwired: 14 in]
      }
      frame "Macro: Initialize" {
        # "Initialization Macro\n(This is called once, when the VI starts)"
        n74 = call <vilib>:"Add State(s) to Queue__jki_lib_state_machine.vi"("State(s) in Front (\"\")"="Data: Initialize\nInitialize Core Data\nUI: Initialize\nUI: Front Panel State >> Open\nMacro: Test", "State(s) in (\"\")"=w229) -> ("States Out"=w228:string)  [unwired: 13 in]
      }
      frame "Macro: Test" {
        # "#Test Macro - Add the sequence \nfor measurments and limits testing here"
        n75 = call <vilib>:"Add State(s) to Queue__jki_lib_state_machine.vi"("State(s) in Front (\"\")"="Limits Test: Read Limits File\nInit: Switch Contactor", "State(s) in (\"\")"=w234) -> ("States Out"=w233:string)  [unwired: 13 in]
      }
      frame "Macro: Limits" {
        # "Do not put any code in this frame.\n(It is a separator no-op. You can make a copy of this frame to create a new Macro frame)"
        n76 = call <vilib>:"Add State(s) to Queue__jki_lib_state_machine.vi"("State(s) in Front (\"\")"="Limits Test: Connect Fail Test\nLimits Test: Connect Test\nLimits Test: UDP Read Test\nLimits Test: 5A Read Test\nLimits Test: Read ROV A Test\nLimits Test: Read ROV B Test\nLimits Test: Read TMS Test\nLimits Test: Read Wait for Start Test\nLimits Test: Read Normal Operation Test\nResults Data: Write Results Data\nMacro: Exit", "State(s) in (\"\")"=w239) -> ("States Out"=w238:string)  [unwired: 13 in]
      }
      frame "Macro: Exit" {
        # "Exit Macro\n(This is called once, when the VI exits)"
        n77 = Unbundle By Name(w246) -> ("Core.Close Panel on Exit?"=w241:bool)
        n78 = call <vilib>:"Conditional State String__jki_lib_state_machine.vi"("Do State(s)?"=w241, "State"="UI: Front Panel State >> Close") -> ("State Out"=w240:string)  [unwired: 7 in]
        n79 = call <vilib>:"Add State(s) to Queue__jki_lib_state_machine.vi"("State(s) in (\"\")"=w240, "State(s) at Back (\"\")"="UI: Uninitialize\nData: Cleanup\nExit") -> ("States Out"=w244:string)  [unwired: 13 in]
        n80 = call <vilib>:"Add State(s) to Queue__jki_lib_state_machine.vi"("State(s) in Front (\"\")"=w244, "State(s) in (\"\")"=w248) -> ("States Out"=w247:string)  [unwired: 13 in]
      }
      frame "---------- Limits Test ----------" {
        # "Template Separator\n(You can make a copy of, or modify, this frame)"
        n81 = call <vilib>:"Add State(s) to Queue__jki_lib_state_machine.vi"("State(s) in (\"\")"=w252) -> ("States Out"=w251:string)  [unwired: 14 in]
      }
      frame "Limits Test: Read Limits File" {
        w258 = ","  # delimiter (\t)
        n82 = Unbundle By Name(w255) -> ("Limits File Path"=w259:path)
        n83 = Current VI's Path "Test Case Path"() -> (path=w263:path)
        n84 = call-poly <vilib>:"Read Delimited Spreadsheet.vi"("file path (dialog if empty)"=w259, "error in (no error)"=w260, "delimiter (\\t)"=w258) -> ("all rows"=w256:string[][], "error out"=w261:errorcluster)  [unwired: 7 in, 4 out]
        n85 = Strip Path(path=w263) -> (name=w262:string)  [unwired: 1 out]
        n86 = call-poly <userlib>:"Strip Path Extension__ogtk.vi"("path"=w262) -> ("root"=w257:string)  [unwired: 1 out]
        n87 = for {
          tunnel: w257 -> [w269]
          tunnel: w256 -> [w267] mode=indexing
          tunnel: [w267] -> w253 mode=indexing if=w266
          n88 = Index Array(array=w267) -> (element=w268:string)  [unwired: 1 in]
          n89 = Equal?(x=w269, y=w268) -> (x = y?=w266:bool)
        }
        n90 = Bundle By Name(cluster=w255, "Test Limits"=w253) -> (w254:T5)
        n91 = call <vilib>:"Add State(s) to Queue__jki_lib_state_machine.vi"("State(s) in (\"\")"=w265) -> ("States Out"=w264:string)  [unwired: 14 in]
      }
      frame "Limits Test: Connect Fail Test" {
        w275 = "Connect Fail Test"  # Sub Test Name
        # "UDP Read Test = if equal to F0 = pass else fail"
        # "#Limits Testing - Add the sub test name for\ntest included in limits file"
        n92 = Unbundle By Name(w274) -> ("Test Limits"=w276:string[][], "Connect Fail"=w280:string)
        n93 = Unbundle By Name(w274) -> ("Results Data Array"=w272:string[][])
        n94 = To Variant(anything=w280) -> (Variant=w277:variant)
        n95 = call "Process Results.vi"("error in (no error)"=w278, "Measurement"=w277, "Test Limits"=w276, "Sub Test Name"=w275) -> ("error out"=w279:errorcluster, "Results Data"=w270:string[])  [unwired: 6 in]
        "Results Data 4" <- w270
        n96 = Build Array (concatenate)(w272, w270) -> (w271:string[][])
        n97 = Bundle By Name(cluster=w274, "Results Data Array"=w271) -> (w273:T5)
        n98 = call <vilib>:"Add State(s) to Queue__jki_lib_state_machine.vi"("State(s) in (\"\")"=w282) -> ("States Out"=w281:string)  [unwired: 14 in]
      }
      frame "Limits Test: Connect Test" {
        w288 = "Connect Test"  # Sub Test Name
        # "UDP Read Test = if equal to F0 = pass else fail"
        # "#Limits Testing - Add the sub test name for\ntest included in limits file"
        n99 = Unbundle By Name(w287) -> ("Results Data Array"=w285:string[][])
        n100 = Unbundle By Name(w287) -> ("Test Limits"=w289:string[][], "Connect"=w293:string)
        n101 = To Variant(anything=w293) -> (Variant=w290:variant)
        n102 = call "Process Results.vi"("error in (no error)"=w291, "Measurement"=w290, "Test Limits"=w289, "Sub Test Name"=w288) -> ("error out"=w292:errorcluster, "Results Data"=w283:string[])  [unwired: 6 in]
        "Results Data 5" <- w283
        n103 = Build Array (concatenate)(w285, w283) -> (w284:string[][])
        n104 = Bundle By Name(cluster=w287, "Results Data Array"=w284) -> (w286:T5)
        n105 = call <vilib>:"Add State(s) to Queue__jki_lib_state_machine.vi"("State(s) in (\"\")"=w295) -> ("States Out"=w294:string)  [unwired: 14 in]
      }
      frame "Limits Test: UDP Read Test" {
        w301 = "UDP Read Test"  # Sub Test Name
        # "UDP Read Test = if equal to F0 = pass else fail"
        # "#Limits Testing - Add the sub test name for\ntest included in limits file"
        n106 = Unbundle By Name(w300) -> ("Results Data Array"=w298:string[][])
        n107 = Unbundle By Name(w300) -> ("Test Limits"=w302:string[][], "UDP Read"=w306:string)
        n108 = To Variant(anything=w306) -> (Variant=w303:variant)
        n109 = call "Process Results.vi"("error in (no error)"=w304, "Measurement"=w303, "Test Limits"=w302, "Sub Test Name"=w301) -> ("error out"=w305:errorcluster, "Results Data"=w296:string[])  [unwired: 6 in]
        "Results Data 2" <- w296
        n110 = Build Array (concatenate)(w298, w296) -> (w297:string[][])
        n111 = Bundle By Name(cluster=w300, "Results Data Array"=w297) -> (w299:T5)
        n112 = call <vilib>:"Add State(s) to Queue__jki_lib_state_machine.vi"("State(s) in (\"\")"=w308) -> ("States Out"=w307:string)  [unwired: 14 in]
      }
      frame "Limits Test: 5A Read Test" {
        w314 = "5A Read Test"  # Sub Test Name
        # "UDP Read Test = if equal to F0 = pass else fail"
        # "#Limits Testing - Add the sub test name for\ntest included in limits file"
        n113 = Unbundle By Name(w313) -> ("Results Data Array"=w311:string[][])
        n114 = Unbundle By Name(w313) -> ("Test Limits"=w315:string[][], "5A Test"=w319:bool)
        n115 = To Variant(anything=w319) -> (Variant=w316:variant)
        n116 = call "Process Results.vi"("error in (no error)"=w317, "Measurement"=w316, "Test Limits"=w315, "Sub Test Name"=w314) -> ("error out"=w318:errorcluster, "Results Data"=w309:string[])  [unwired: 6 in]
        "Results Data 3" <- w309
        n117 = Build Array (concatenate)(w311, w309) -> (w310:string[][])
        n118 = Bundle By Name(cluster=w313, "Results Data Array"=w310) -> (w312:T5)
        n119 = call <vilib>:"Add State(s) to Queue__jki_lib_state_machine.vi"("State(s) in (\"\")"=w321) -> ("States Out"=w320:string)  [unwired: 14 in]
      }
      frame "Limits Test: Read ROV A Test" {
        w327 = "Read ROV A Test"  # Sub Test Name
        # "UDP Read Test = if equal to F0 = pass else fail"
        # "#Limits Testing - Add the sub test name for\ntest included in limits file"
        n120 = Unbundle By Name(w326) -> ("Test Limits"=w328:string[][], "Read ROV A"=w332:string)
        n121 = Unbundle By Name(w326) -> ("Results Data Array"=w324:string[][])
        n122 = To Variant(anything=w332) -> (Variant=w329:variant)
        n123 = call "Process Results.vi"("error in (no error)"=w330, "Measurement"=w329, "Test Limits"=w328, "Sub Test Name"=w327) -> ("error out"=w331:errorcluster, "Results Data"=w322:string[])  [unwired: 6 in]
        "Results Data 6" <- w322
        n124 = Build Array (concatenate)(w324, w322) -> (w323:string[][])
        n125 = Bundle By Name(cluster=w326, "Results Data Array"=w323) -> (w325:T5)
        n126 = call <vilib>:"Add State(s) to Queue__jki_lib_state_machine.vi"("State(s) in (\"\")"=w334) -> ("States Out"=w333:string)  [unwired: 14 in]
      }
      frame "Limits Test: Read ROV B Test" {
        w340 = "Read ROV B Test"  # Sub Test Name
        # "UDP Read Test = if equal to F0 = pass else fail"
        # "#Limits Testing - Add the sub test name for\ntest included in limits file"
        n127 = Unbundle By Name(w339) -> ("Test Limits"=w341:string[][], "Read ROV B"=w345:string)
        n128 = Unbundle By Name(w339) -> ("Results Data Array"=w337:string[][])
        n129 = To Variant(anything=w345) -> (Variant=w342:variant)
        n130 = call "Process Results.vi"("error in (no error)"=w343, "Measurement"=w342, "Test Limits"=w341, "Sub Test Name"=w340) -> ("error out"=w344:errorcluster, "Results Data"=w335:string[])  [unwired: 6 in]
        "Results Data 7" <- w335
        n131 = Build Array (concatenate)(w337, w335) -> (w336:string[][])
        n132 = Bundle By Name(cluster=w339, "Results Data Array"=w336) -> (w338:T5)
        n133 = call <vilib>:"Add State(s) to Queue__jki_lib_state_machine.vi"("State(s) in (\"\")"=w347) -> ("States Out"=w346:string)  [unwired: 14 in]
      }
      frame "Limits Test: Read TMS Test" {
        w353 = "Read TMS Test"  # Sub Test Name
        # "UDP Read Test = if equal to F0 = pass else fail"
        # "#Limits Testing - Add the sub test name for\ntest included in limits file"
        n134 = Unbundle By Name(w352) -> ("Results Data Array"=w350:string[][])
        n135 = Unbundle By Name(w352) -> ("Test Limits"=w354:string[][], "Read TMS"=w358:string)
        n136 = To Variant(anything=w358) -> (Variant=w355:variant)
        n137 = call "Process Results.vi"("error in (no error)"=w356, "Measurement"=w355, "Test Limits"=w354, "Sub Test Name"=w353) -> ("error out"=w357:errorcluster, "Results Data"=w348:string[])  [unwired: 6 in]
        "Results Data 8" <- w348
        n138 = Build Array (concatenate)(w350, w348) -> (w349:string[][])
        n139 = Bundle By Name(cluster=w352, "Results Data Array"=w349) -> (w351:T5)
        n140 = call <vilib>:"Add State(s) to Queue__jki_lib_state_machine.vi"("State(s) in (\"\")"=w360) -> ("States Out"=w359:string)  [unwired: 14 in]
      }
      frame "Limits Test: Read Wait for Start Test" {
        w366 = "Read Wait for Start Test"  # Sub Test Name
        # "UDP Read Test = if equal to F0 = pass else fail"
        # "#Limits Testing - Add the sub test name for\ntest included in limits file"
        n141 = Unbundle By Name(w365) -> ("Test Limits"=w367:string[][], "Read Wait for Start"=w371:string)
        n142 = Unbundle By Name(w365) -> ("Results Data Array"=w363:string[][])
        n143 = To Variant(anything=w371) -> (Variant=w368:variant)
        n144 = call "Process Results.vi"("error in (no error)"=w369, "Measurement"=w368, "Test Limits"=w367, "Sub Test Name"=w366) -> ("error out"=w370:errorcluster, "Results Data"=w361:string[])  [unwired: 6 in]
        "Results Data 9" <- w361
        n145 = Build Array (concatenate)(w363, w361) -> (w362:string[][])
        n146 = Bundle By Name(cluster=w365, "Results Data Array"=w362) -> (w364:T5)
        n147 = call <vilib>:"Add State(s) to Queue__jki_lib_state_machine.vi"("State(s) in (\"\")"=w373) -> ("States Out"=w372:string)  [unwired: 14 in]
      }
      frame "Limits Test: Read Normal Operation Test" {
        w379 = "Read Normal Operation Test"  # Sub Test Name
        # "UDP Read Test = if equal to F0 = pass else fail"
        # "#Limits Testing - Add the sub test name for\ntest included in limits file"
        n148 = Unbundle By Name(w378) -> ("Test Limits"=w380:string[][], "Read Normal Operation"=w384:string)
        n149 = Unbundle By Name(w378) -> ("Results Data Array"=w376:string[][])
        n150 = To Variant(anything=w384) -> (Variant=w381:variant)
        n151 = call "Process Results.vi"("error in (no error)"=w382, "Measurement"=w381, "Test Limits"=w380, "Sub Test Name"=w379) -> ("error out"=w383:errorcluster, "Results Data"=w374:string[])  [unwired: 6 in]
        "Results Data 10" <- w374
        n152 = Build Array (concatenate)(w376, w374) -> (w375:string[][])
        n153 = Bundle By Name(cluster=w378, "Results Data Array"=w375) -> (w377:T5)
        n154 = call <vilib>:"Add State(s) to Queue__jki_lib_state_machine.vi"("State(s) in (\"\")"=w386) -> ("States Out"=w385:string)  [unwired: 14 in]
      }
      frame "---------- Results Data ----------" {
        # "Template Separator\n(You can make a copy of, or modify, this frame)"
        n155 = call <vilib>:"Add State(s) to Queue__jki_lib_state_machine.vi"("State(s) in (\"\")"=w390) -> ("States Out"=w389:string)  [unwired: 14 in]
      }
      frame "Results Data: Write Results Data" {
        w392 = ","  # delimiter (\t)
        w393 = TRUE  # append to file? (new file:F)
        n156 = Unbundle By Name(w395) -> ("Results File Path"=w394:path, "Results Data Array"=w391:string[][])
        "Results Data Array" <- w391
        n157 = call-poly <vilib>:"Write Delimited Spreadsheet.vi"("file path (dialog if empty)"=w394, "2D data"=w391, "append to file? (new file:F)"=w393, "error in (no error)"=w396, "delimiter (\\t)"=w392) -> ("error out"=w397:errorcluster)  [unwired: 9 in, 1 out]
        n158 = call <vilib>:"Add State(s) to Queue__jki_lib_state_machine.vi"("State(s) in (\"\")"=w399) -> ("States Out"=w398:string)  [unwired: 14 in]
      }
      frame "---------- Init ----------" {
        # "Template Separator\n(You can make a copy of, or modify, this frame)"
        n159 = call <vilib>:"Add State(s) to Queue__jki_lib_state_machine.vi"("State(s) in (\"\")"=w403) -> ("States Out"=w402:string)  [unwired: 14 in]
      }
      frame "Init: Switch Contactor" {
        # "Template Separator\n(You can make a copy of, or modify, this frame)"
        # "User must set IP address to match this given one"
        n160 = call-poly <vilib>:"DAQmx Create Virtual Channel.vi"("lines"=tag "6525/port0/line0", "error in"=w412) -> ("task out"=w415:refnum<k21>, "error out"=w414:errorcluster)  [unwired: 12 in]
        n161 = call <vilib>:"DAQmx Start Task.vi"("task/channels in"=w415, "error in"=w414) -> ("task out"=w410:refnum<k21>, "error out"=w411:errorcluster)  [unwired: 12 in]
        n162 = call-poly <vilib>:"DAQmx Write.vi"("task/channels in"=w410, "data"=bool[] [TRUE], "error in"=w411) -> ("task out"=w405:refnum<k21>, "error out"=w409:errorcluster)  [unwired: 10 in, 1 out]
        n163 = call <vilib>:"DAQmx Stop Task.vi"("task/channels in"=w405, "error in"=w409) -> ("task out"=w406:refnum<k21>, "error out"=w408:errorcluster)  [unwired: 12 in]
        n164 = call <vilib>:"DAQmx Clear Task.vi"("task in"=w406, "error in"=w408) -> ("error out"=w407:errorcluster)  [unwired: 13 in]
        n165 = call <vilib>:"Add State(s) to Queue__jki_lib_state_machine.vi"("State(s) in Front (\"\")"="Init: Set IP Address" ("State(s) in Front (\"\")"), "State(s) in (\"\")"=w419) -> ("States Out"=w418:string)  [unwired: 13 in]
      }
      frame "Init: Set IP Address" {
        # "Template Separator\n(You can make a copy of, or modify, this frame)"
        # "User must set IP address to match this given one"
        n166 = One Button Dialog(message="Make your IP Address 192.168.201.22", button name ("OK")="Done") -> ()  [unwired: 1 out]
        n167 = call <vilib>:"Add State(s) to Queue__jki_lib_state_machine.vi"("State(s) in Front (\"\")"="Init: UDP Open" ("State(s) in Front (\"\")"), "State(s) in (\"\")"=w426) -> ("States Out"=w425:string)  [unwired: 13 in]
      }
      frame "Init: UDP Open" {
        # "If this changes \nchange on CONNECT command as well!"
        # "User must enter their PC IP address"
        # "Open UDP read to RIB box"
        # "Template Separator\n(You can make a copy of, or modify, this frame)"
        # "Open UDP linking to RIB Box."
        n168 = String To IP(1:"192.168.201.22" ("name")) -> (0:w436:u32)
        n169 = UDP Open(7:w436, 8:w435, 11:u16 54321 ("port")) -> (port=w429:refnum<k16>, 0:w431:errorcluster)  [unwired: 2 in, 1 out]
        n170 = call "FGV - Initialise.vi"("Enum"=FGV_-_Enum."Open UDP", "connection ID"=w429, "Error In"=w431) -> ("Error Out"=w430:errorcluster)  [unwired: 9 in, 3 out]
        n171 = Bundle By Name(cluster=w434, "connection ID"=w429) -> (w433:T5)
        n172 = call <vilib>:"Add State(s) to Queue__jki_lib_state_machine.vi"("State(s) in Front (\"\")"="Init: I2C Open" ("State(s) in Front (\"\")"), "State(s) in (\"\")"=w439) -> ("States Out"=w438:string)  [unwired: 13 in]
      }
      frame "Init: I2C Open" {
        # "Template Separator\n(You can make a copy of, or modify, this frame)"
        n173 = call "FGV - Initialise.vi"("Enum"=FGV_-_Enum."Get Data", "Error In"=w442) -> ("task out"=w441:refnum<k21>, "Error Out"=w443:errorcluster)  [unwired: 10 in, 2 out]
        n174 = Bundle By Name(cluster=w446, "task out"=w441) -> (w445:T5)
        n175 = call <vilib>:"Add State(s) to Queue__jki_lib_state_machine.vi"("State(s) in Front (\"\")"="Init: UPD Connect Fail" ("State(s) in Front (\"\")"), "State(s) in (\"\")"=w448) -> ("States Out"=w447:string)  [unwired: 13 in]
      }
      frame "Init: UPD Connect Fail" {
        # "Send CONNECT command to RIB Box"
        # "IP for RIB Box is set"
        # "Data"
        # "Length"
        # "ID"
        # "Target"
        # "Type"
        # "Pkt ID"
        # "CONNECT"
        # "Template Separator\n(You can make a copy of, or modify, this frame)"
        n176 = Unbundle By Name(w454) -> ("connection ID"=w453:refnum<k16>)
        n177 = Build Array(u8 91 ("element"), u8 1 ("element"), u8 9 ("element"), u8 1 ("element"), u8 5 ("element"), u8 192 ("element"), u8 168 ("element"), u8 201 ("element"), u8 255 ("element")) -> (w469:u8[])
        n178 = Byte Array To String(unsigned byte array=w469) -> (string=w470:string)
        n179 = String To IP(1:"192.168.201.21" ("name")) -> (0:w458:u32)
        n180 = UDP Write(address=w458, port or service name=u16 54321, connection ID=w453, data in=w470, 8:w455, 9:1000 ("timeout ms (25000)")) -> (error out=w450:errorcluster, 3:w452:refnum<k16>)
        n181 = Bundle By Name(cluster=w454, "connection ID"=w452) -> (w456:T5)
        n182 = Wait (ms)(milliseconds to wait=u32 100) -> ()  [unwired: 1 out]
        n183 = call <vilib>:"Add State(s) to Queue__jki_lib_state_machine.vi"("State(s) in Front (\"\")"="Init: Read Connect Fail" ("State(s) in Front (\"\")"), "State(s) in (\"\")"=w473) -> ("States Out"=w472:string)  [unwired: 13 in]
      }
      frame "Init: Read Connect Fail" {
        # "Read UDP if equal to F0 test complete if not check if timer has elapsed."
        # "#56 = didnt read before the timeout"
        # "Template Separator\n(You can make a copy of, or modify, this frame)"
        n184 = Unbundle By Name(w495) -> ("connection ID"=w496:refnum<k16>)
        n185 = UDP Read(connection ID=w496, timeout ms (25000)=10, 8:w497) -> (data out=w486:string, error out=w491:errorcluster, 3:w488:refnum<k16>)  [unwired: 1 in, 2 out]
        n186 = String To Byte Array(string=w486) -> (unsigned byte array=w493:u8[])
        n187 = Number To Hexadecimal String(2:w493) -> (0:w478:string[])  [unwired: 1 in]
        n188 = Index Array(array=w478, index #1=0 ("index")) -> (element #1=w480:string, element #2=w484:string, element #3=w483:string, element #4=w482:string, element #5=w481:string, element #6=w477:string, element #7=w476:string, element #8=w475:string, element #9=w474:string)  [unwired: 8 in]
        n189 = Concatenate Strings(w480, w484, w483, w482, w481, w477, w476, w475, w474) -> (w479:string)
        n190 = call <vilib>:"Clear Errors.vi"("error in (no error)"=w491, "specific error code to clear (0: all)"=56) -> ("error out"=w490:errorcluster)  [unwired: 4 in, 1 out]
        n191 = Bundle By Name(cluster=w495, "connection ID"=w488, "Connect Fail"=w479) -> (w494:T5)
        n192 = call <vilib>:"Add State(s) to Queue__jki_lib_state_machine.vi"("State(s) in Front (\"\")"="Init: UPD Connect" ("State(s) in Front (\"\")"), "State(s) in (\"\")"=w499) -> ("States Out"=w498:string)  [unwired: 13 in]
      }
      frame "Init: UPD Connect" {
        # "Length Wrong to froce a fail!"
        # "Send CONNECT command to RIB Box"
        # "IP for RIB Box is set"
        # "Data"
        # "Length"
        # "ID"
        # "Target"
        # "Type"
        # "Pkt ID"
        # "CONNECT"
        # "Template Separator\n(You can make a copy of, or modify, this frame)"
        n193 = Unbundle By Name(w505) -> ("connection ID"=w504:refnum<k16>)
        n194 = Build Array(u8 91 ("element"), u8 1 ("element"), u8 9 ("element"), u8 1 ("element"), u8 4 ("element"), u8 192 ("element"), u8 168 ("element"), u8 201 ("element"), u8 22 ("element")) -> (w520:u8[])
        n195 = Byte Array To String(unsigned byte array=w520) -> (string=w521:string)
        n196 = String To IP(1:"192.168.201.21" ("name")) -> (0:w509:u32)
        n197 = UDP Write(address=w509, port or service name=u16 54321, connection ID=w504, data in=w521, 8:w506, 9:1000 ("timeout ms (25000)")) -> (error out=w501:errorcluster, 3:w503:refnum<k16>)
        n198 = Bundle By Name(cluster=w505, "connection ID"=w503) -> (w507:T5)
        n199 = Wait (ms)(milliseconds to wait=u32 100) -> ()  [unwired: 1 out]
        n200 = call <vilib>:"Add State(s) to Queue__jki_lib_state_machine.vi"("State(s) in Front (\"\")"="Init: Read Connect" ("State(s) in Front (\"\")"), "State(s) in (\"\")"=w524) -> ("States Out"=w523:string)  [unwired: 13 in]
      }
      frame "Init: Read Connect" {
        # "Read UDP if equal to F0 test complete if not check if timer has elapsed."
        # "#56 = didnt read before the timeout"
        # "Template Separator\n(You can make a copy of, or modify, this frame)"
        n201 = Unbundle By Name(w546) -> ("connection ID"=w547:refnum<k16>)
        n202 = UDP Read(connection ID=w547, timeout ms (25000)=10, 8:w548) -> (data out=w537:string, error out=w543:errorcluster, 3:w540:refnum<k16>)  [unwired: 1 in, 2 out]
        n203 = String To Byte Array(string=w537) -> (unsigned byte array=w538:u8[])
        n204 = Number To Hexadecimal String(2:w538) -> (0:w526:string[])  [unwired: 1 in]
        n205 = Index Array(array=w526, index #1=0 ("index")) -> (element #1=w531:string, element #2=w535:string, element #3=w534:string, element #4=w533:string, element #5=w532:string, element #6=w530:string, element #7=w529:string, element #8=w528:string, element #9=w527:string)  [unwired: 8 in]
        n206 = Concatenate Strings(w531, w535, w534, w533, w532, w530, w529, w528, w527) -> (w525:string)
        n207 = call <vilib>:"Clear Errors.vi"("error in (no error)"=w543, "specific error code to clear (0: all)"=56) -> ("error out"=w542:errorcluster)  [unwired: 4 in, 1 out]
        n208 = Bundle By Name(cluster=w546, "connection ID"=w540, "Connect"=w525) -> (w545:T5)
        n209 = call <vilib>:"Add State(s) to Queue__jki_lib_state_machine.vi"("State(s) in Front (\"\")"="Init: Start Timer" ("State(s) in Front (\"\")"), "State(s) in (\"\")"=w550) -> ("States Out"=w549:string)  [unwired: 13 in]
      }
      frame "Init: Start Timer" {
        # "Start 10 second timer"
        # "Template Separator\n(You can make a copy of, or modify, this frame)"
        n210 = call "Timer.vi"("error in (no error)"=w557, "Enum"=T4."Start Timer") -> ("error out"=w556:errorcluster)  [unwired: 6 in, 3 out]
        n211 = property on="Timeout (Read UDP)" class="Slide (strict)"(error in=w556, "Value"=0.0 ("Horizontal Pointer Slide"), "Scale.Maximum"=20.0 ("Target Time"), "Scale.Minimum"=0.0 ("Scale.Range:Minimum")) -> (error out=w552:errorcluster)  [unwired: 1 in, 1 out]
        n212 = call <vilib>:"Add State(s) to Queue__jki_lib_state_machine.vi"("State(s) in Front (\"\")"="Init: UPD Enable UPS" ("State(s) in Front (\"\")"), "State(s) in (\"\")"=w561) -> ("States Out"=w560:string)  [unwired: 13 in]
      }
      frame "Init: UPD Enable UPS" {
        # "Send Enable UPS command to RIB Box"
        # "ENABLE UPS"
        # "Template Separator\n(You can make a copy of, or modify, this frame)"
        n213 = Unbundle By Name(w565) -> ("connection ID"=w564:refnum<k16>)
        n214 = Build Array(u8 91 ("element"), u8 1 ("element"), u8 9 ("element"), u8 112 ("element"), u8 1 ("element"), u8 1 ("element")) -> (w579:u8[])
        n215 = String To IP(1:"192.168.201.21" ("name")) -> (0:w572:u32)
        n216 = Byte Array To String(unsigned byte array=w579) -> (string=w573:string)
        n217 = UDP Write(address=w572, port or service name=u16 54321, connection ID=w564, data in=w573, 8:w567, 9:1000 ("timeout ms (25000)")) -> (error out=w562:errorcluster, 3:w568:refnum<k16>)
        n218 = Bundle By Name(cluster=w565, "connection ID"=w568) -> (w569:T5)
        n219 = call <vilib>:"Add State(s) to Queue__jki_lib_state_machine.vi"("State(s) in Front (\"\")"="Init: Read UDP" ("State(s) in Front (\"\")"), "State(s) in (\"\")"=w582) -> ("States Out"=w581:string)  [unwired: 13 in]
      }
      frame "Init: Read UDP" {
        # "Read UDP if equal to F0 test complete if not check if timer has elapsed."
        # "#56 = didnt read before the timeout"
        # "Template Separator\n(You can make a copy of, or modify, this frame)"
        n220 = Unbundle By Name(w600) -> ("connection ID"=w601:refnum<k16>)
        n221 = UDP Read(connection ID=w601, timeout ms (25000)=10, 8:w602) -> (data out=w588:string, error out=w587:errorcluster, 3:w583:refnum<k16>)  [unwired: 1 in, 2 out]
        n222 = String Subset(string=w588, offset (0)=81 ("offset (0) 2"), length (rest)=1 ("length (rest) 2")) -> (substring=w595:string)
        n223 = String To Byte Array(string=w595) -> (unsigned byte array=w598:u8[])
        n224 = Number To Hexadecimal String(2:w598) -> (0:w597:string[])  [unwired: 1 in]
        n225 = Index Array(array=w597, index=0) -> (element=w584:string)
        n226 = call <vilib>:"Clear Errors.vi"("error in (no error)"=w587, "specific error code to clear (0: all)"=56) -> ("error out"=w586:errorcluster)  [unwired: 4 in, 1 out]
        n227 = Equal?(x=w584, y="F0") -> (x = y?=w592:bool)
        n228 = Bundle By Name(cluster=w600, "connection ID"=w583, "UDP Read"=w584) -> (w599:T5)
        n229 = call-poly <vilib>:"Select State(s)__jki_lib_state_machine.vi"("State(s) if True (\"\")"="Init: Start Timer (5A)" ("State(s) if True (\"\")"), "Select"=w592, "State(s) if False (\"\")"="Init: Elapsed Timer" ("State(s) if False (\"\")")) -> ("States Out"=w590:string)  [unwired: 12 in]
        n230 = call <vilib>:"Add State(s) to Queue__jki_lib_state_machine.vi"("State(s) in Front (\"\")"=w590, "State(s) in (\"\")"=w606) -> ("States Out"=w605:string)  [unwired: 13 in]
      }
      frame "Init: Elapsed Timer" {
        # "check if timer elased - if TRUE end test if FALSE read again."
        # "Template Separator\n(You can make a copy of, or modify, this frame)"
        # "Check to see if the timer has elpased."
        n231 = call "Timer.vi"("error in (no error)"=w614, "Target Time"=20.0, "Enum"=T4."Get Time") -> ("error out"=w613:errorcluster, "Time Elapsed?"=w610:bool, "Elapsed Time"=→"Timeout (Read UDP)":dbl)  [unwired: 5 in, 1 out]
        n232 = call-poly <vilib>:"Select State(s)__jki_lib_state_machine.vi"("State(s) if True (\"\")"="Init: Start Timer (5A)" ("State(s) if True (\"\")"), "Select"=w610, "State(s) if False (\"\")"="Init: Read UDP" ("State(s) if False (\"\")")) -> ("States Out"=w609:string)  [unwired: 12 in]
        n233 = call <vilib>:"Add State(s) to Queue__jki_lib_state_machine.vi"("State(s) in Front (\"\")"=w609, "State(s) in (\"\")"=w618) -> ("States Out"=w617:string)  [unwired: 13 in]
      }
      frame "Init: Start Timer (5A)" {
        # "Start 5 second timer"
        # "Template Separator\n(You can make a copy of, or modify, this frame)"
        n234 = call "Timer.vi"("error in (no error)"=w625, "Enum"=T4."Start Timer") -> ("error out"=w620:errorcluster)  [unwired: 6 in, 3 out]
        n235 = property on="Timeout (5A)" class="Slide (strict)"(error in=w620, "Value"=0.0 ("Horizontal Pointer Slide"), "Scale.Maximum"=5.0 ("Target Time"), "Scale.Minimum"=0.0 ("Scale.Range:Minimum")) -> (error out=w619:errorcluster)  [unwired: 1 in, 1 out]
        n236 = call <vilib>:"Add State(s) to Queue__jki_lib_state_machine.vi"("State(s) in Front (\"\")"="Init: Check 5A" ("State(s) in Front (\"\")"), "State(s) in (\"\")"=w629) -> ("States Out"=w628:string)  [unwired: 13 in]
      }
      frame "Init: Check 5A" {
        # "Template Copyright © 2024 JKI - http://jki.net/state-machine"
        # "Measure 5A from the 6525. If it can be read test complete else the timer progress is made."
        n237 = Unbundle By Name(w645) -> ("task out"=w636:refnum<k21>)
        n238 = call-poly <vilib>:"DAQmx Read.vi"("task/channels in"=w636, "error in"=w635) -> ("task out"=w630:refnum<k21>, "data"=w643:bool[], "error out"=w634:errorcluster)  [unwired: 11 in]
        n239 = Equal?(x=bool[] [TRUE, TRUE, TRUE, TRUE, FALSE], y=w643) -> (x = y?=w638:bool[])
        n240 = Array To Cluster(array=w638) -> (cluster=w639:T7)
        n241 = Unbundle(w639) -> ("[0]"=w640:bool, "[1]"=w641:bool, "[2]"=w642:bool, "[3]"=w632:bool)  [unwired: 5 out]
        n242 = Compound Arithmetic op=AND(w640, w641, w642, w632) -> (w631:bool)
        "5A Test" <- w631
        n243 = Bundle By Name(cluster=w645, "task out"=w630, "5A Test"=w631) -> (w644:T5)
        n244 = call-poly <vilib>:"Select State(s)__jki_lib_state_machine.vi"("State(s) if True (\"\")"="Init: Enable ROV A, ROV B and TMS" ("State(s) if True (\"\")"), "Select"=w631, "State(s) if False (\"\")"="Init: Elapsed Timer (5A)" ("State(s) if False (\"\")")) -> ("States Out"=w646:string)  [unwired: 12 in]
        n245 = call <vilib>:"Add State(s) to Queue__jki_lib_state_machine.vi"("State(s) in Front (\"\")"=w646, "State(s) in (\"\")"=w649) -> ("States Out"=w648:string)  [unwired: 13 in]
      }
      frame "Init: Elapsed Timer (5A)" {
        # "check if timer elased - if TRUE end test if FALSE read again."
        # "Template Separator\n(You can make a copy of, or modify, this frame)"
        n246 = call "Timer.vi"("error in (no error)"=w657, "Target Time"=5.0, "Enum"=T4."Get Time") -> ("error out"=w656:errorcluster, "Time Elapsed?"=w653:bool, "Elapsed Time"=→"Timeout (5A)":dbl)  [unwired: 5 in, 1 out]
        n247 = call-poly <vilib>:"Select State(s)__jki_lib_state_machine.vi"("State(s) if True (\"\")"="Init: Enable ROV A, ROV B and TMS" ("State(s) if True (\"\")"), "Select"=w653, "State(s) if False (\"\")"="Init: Check 5A" ("State(s) if False (\"\")")) -> ("States Out"=w652:string)  [unwired: 12 in]
        n248 = call <vilib>:"Add State(s) to Queue__jki_lib_state_machine.vi"("State(s) in Front (\"\")"=w652, "State(s) in (\"\")"=w661) -> ("States Out"=w660:string)  [unwired: 13 in]
      }
      frame "Init: Enable ROV A, ROV B and TMS" {
        w690 = u16 54321 ("port or service name")
        # "Data"
        # "Length"
        # "ID"
        # "Target"
        # "Type"
        # "Pkt ID"
        # "Data"
        # "Length"
        # "ID"
        # "Target"
        # "Type"
        # "Pkt ID"
        # "Data"
        # "Length"
        # "ID"
        # "Target"
        # "Type"
        # "Pkt ID"
        # "Send Enable UPS command to RIB Box"
        # "Template Separator\n(You can make a copy of, or modify, this frame)"
        n249 = Unbundle By Name(w670) -> ("connection ID"=w669:refnum<k16>)
        n250 = Build Array(u8 91 ("element"), u8 1 ("element"), u8 9 ("element"), u8 105 ("element"), u8 1 ("element"), u8 1 ("element")) -> (w700:u8[])
        n251 = Byte Array To String(unsigned byte array=w700) -> (string=w697:string)
        n252 = String To IP(1:"192.168.201.21" ("name")) -> (0:w703:u32)
        n253 = UDP Write(address=w703, port or service name=w690, connection ID=w669, data in=w697, 8:w673, 9:1000 ("timeout ms (25000)")) -> (error out=w662:errorcluster, 3:w666:refnum<k16>)
        n254 = Build Array(u8 91 ("element"), u8 1 ("element"), u8 9 ("element"), u8 106 ("element"), u8 1 ("element"), u8 1 ("element")) -> (w701:u8[])
        n255 = Byte Array To String(unsigned byte array=w701) -> (string=w698:string)
        n256 = UDP Write(address=w703, port or service name=w690, connection ID=w666, data in=w698, 8:w662, 9:1000 ("timeout ms (25000)")) -> (error out=w672:errorcluster, 3:w667:refnum<k16>)
        n257 = Build Array(u8 91 ("element"), u8 1 ("element"), u8 9 ("element"), u8 107 ("element"), u8 1 ("element"), u8 1 ("element")) -> (w702:u8[])
        n258 = Byte Array To String(unsigned byte array=w702) -> (string=w699:string)
        n259 = UDP Write(address=w703, port or service name=w690, connection ID=w667, data in=w699, 8:w672, 9:1000 ("timeout ms (25000)")) -> (error out=w665:errorcluster, 3:w671:refnum<k16>)
        n260 = Bundle By Name(cluster=w670, "connection ID"=w671) -> (w704:T5)
        n261 = call <userlib>:"Wait (ms)__ogtk.vi"("error in (no error)"=w665, "milliseconds to wait"=u32 1000) -> ("error out"=w664:errorcluster)  [unwired: 8 in, 1 out]
        n262 = call <vilib>:"Add State(s) to Queue__jki_lib_state_machine.vi"("State(s) in Front (\"\")"="Init: Set Command" ("State(s) in Front (\"\")"), "State(s) in (\"\")"=w706) -> ("States Out"=w705:string)  [unwired: 13 in]
      }
      frame "Init: Set Command" {
        # "RIB Box IP"
        # "Data"
        # "Length"
        # "ID"
        # "Target"
        # "Type"
        # "Pkt ID"
        # "SET"
        # "Template Separator\n(You can make a copy of, or modify, this frame)"
        n263 = Unbundle By Name(w725) -> ("connection ID"=w712:refnum<k16>)
        n264 = Build Array(u8 91 ("element"), u8 1 ("element"), u8 9 ("element"), u8 108 ("element"), u8 0 ("element")) -> (w723:u8[])
        n265 = Byte Array To String(unsigned byte array=w723) -> (string=w724:string)
        n266 = String To IP(1:"192.168.201.21" ("name")) -> (0:w716:u32)
        n267 = UDP Write(address=w716, port or service name=u16 54321, connection ID=w712, data in=w724, 8:w714, 9:1000 ("timeout ms (25000)")) -> (error out=w709:errorcluster, 3:w713:refnum<k16>)
        n268 = Bundle By Name(cluster=w725, "connection ID"=w713) -> (w726:T5)
        n269 = call <userlib>:"Wait (ms)__ogtk.vi"("error in (no error)"=w709, "milliseconds to wait"=u32 1000) -> ("error out"=w708:errorcluster)  [unwired: 8 in, 1 out]
        n270 = call <vilib>:"Add State(s) to Queue__jki_lib_state_machine.vi"("State(s) in Front (\"\")"="Init: Start Timer (ROV A)" ("State(s) in Front (\"\")"), "State(s) in (\"\")"=w728) -> ("States Out"=w727:string)  [unwired: 13 in]
      }
      frame "Init: Start Timer (ROV A)" {
        # "Start 10 second timer"
        # "Template Separator\n(You can make a copy of, or modify, this frame)"
        n271 = call "Timer.vi"("error in (no error)"=w735, "Enum"=T4."Start Timer") -> ("error out"=w734:errorcluster)  [unwired: 6 in, 3 out]
        n272 = property on="Timeout (Read States)" class="Slide (strict)"(error in=w734, "Value"=0.0 ("Horizontal Pointer Slide"), "Scale.Maximum"=15.0 ("Target Time"), "Scale.Minimum"=0.0 ("Scale.Range:Minimum")) -> (error out=w730:errorcluster)  [unwired: 1 in, 1 out]
        n273 = call <vilib>:"Add State(s) to Queue__jki_lib_state_machine.vi"("State(s) in Front (\"\")"="Init: Read ROV A State" ("State(s) in Front (\"\")"), "State(s) in (\"\")"=w739) -> ("States Out"=w738:string)  [unwired: 13 in]
      }
      frame "Init: Read ROV A State" {
        # "Read UDP if equal to F0 test complete if not check if timer has elapsed."
        # "#56 = didnt read before the timeout"
        # "Template Separator\n(You can make a copy of, or modify, this frame)"
        n274 = Unbundle By Name(w749) -> ("connection ID"=w759:refnum<k16>)
        n275 = UDP Read(connection ID=w759, timeout ms (25000)=1, 8:w746) -> (data out=w753:string, error out=w752:errorcluster, 3:w750:refnum<k16>)  [unwired: 1 in, 2 out]
        n276 = String Subset(string=w753, offset (0)=17 ("offset (0) 2"), length (rest)=1 ("length (rest) 2")) -> (substring=w755:string)
        n277 = String To Byte Array(string=w755) -> (unsigned byte array=w758:u8[])
        n278 = Number To Hexadecimal String(2:w758) -> (0:w757:string[])  [unwired: 1 in]
        n279 = Index Array(array=w757, index=0) -> (element=w740:string)
        "element" <- w740
        n280 = Equal?(x=w740, y="C") -> (x = y?=w741:bool)
        "ROV A Enabled" <- w741
        n281 = call <vilib>:"Clear Errors.vi"("error in (no error)"=w752, "specific error code to clear (0: all)"=56) -> ("error out"=w747:errorcluster)  [unwired: 4 in, 1 out]
        n282 = Bundle By Name(cluster=w749, "connection ID"=w750, "Read ROV A"=w740) -> (w748:T5)
        n283 = call-poly <vilib>:"Select State(s)__jki_lib_state_machine.vi"("State(s) if True (\"\")"="Init: Start Timer (ROV B)" ("State(s) if True (\"\")"), "Select"=w741, "State(s) if False (\"\")"="Init: Elapsed Timer (ROV A)" ("State(s) if False (\"\")")) -> ("States Out"=w742:string)  [unwired: 12 in]
        n284 = call <vilib>:"Add State(s) to Queue__jki_lib_state_machine.vi"("State(s) in Front (\"\")"=w742, "State(s) in (\"\")"=w763) -> ("States Out"=w762:string)  [unwired: 13 in]
      }
      frame "Init: Elapsed Timer (ROV A)" {
        # "check if timer elased - if TRUE end test if FALSE read again."
        # "Template Separator\n(You can make a copy of, or modify, this frame)"
        # "Check to see if the timer has elpased."
        n285 = call "Timer.vi"("error in (no error)"=w771, "Target Time"=15.0, "Enum"=T4."Get Time") -> ("error out"=w770:errorcluster, "Time Elapsed?"=w767:bool, "Elapsed Time"=→"Timeout (Read States)":dbl)  [unwired: 5 in, 1 out]
        n286 = call-poly <vilib>:"Select State(s)__jki_lib_state_machine.vi"("State(s) if True (\"\")"="Init: Start Timer (ROV B)" ("State(s) if True (\"\")"), "Select"=w767, "State(s) if False (\"\")"="Init: Read ROV A State" ("State(s) if False (\"\")")) -> ("States Out"=w766:string)  [unwired: 12 in]
        n287 = call <vilib>:"Add State(s) to Queue__jki_lib_state_machine.vi"("State(s) in Front (\"\")"=w766, "State(s) in (\"\")"=w775) -> ("States Out"=w774:string)  [unwired: 13 in]
      }
      frame "Init: Start Timer (ROV B)" {
        # "Start 10 second timer"
        # "Template Separator\n(You can make a copy of, or modify, this frame)"
        n288 = call "Timer.vi"("error in (no error)"=w782, "Enum"=T4."Start Timer") -> ("error out"=w781:errorcluster)  [unwired: 6 in, 3 out]
        n289 = property on="Timeout (Read States) 2" class="Slide (strict)"(error in=w781, "Value"=0.0 ("Horizontal Pointer Slide"), "Scale.Maximum"=10.0 ("Target Time"), "Scale.Minimum"=0.0 ("Scale.Range:Minimum")) -> (error out=w777:errorcluster)  [unwired: 1 in, 1 out]
        n290 = call <vilib>:"Add State(s) to Queue__jki_lib_state_machine.vi"("State(s) in Front (\"\")"="Init: Read ROV B State" ("State(s) in Front (\"\")"), "State(s) in (\"\")"=w786) -> ("States Out"=w785:string)  [unwired: 13 in]
      }
      frame "Init: Read ROV B State" {
        # "Read UDP if equal to F0 test complete if not check if timer has elapsed."
        # "#56 = didnt read before the timeout"
        # "Template Separator\n(You can make a copy of, or modify, this frame)"
        n291 = Unbundle By Name(w793) -> ("connection ID"=w806:refnum<k16>)
        n292 = UDP Read(connection ID=w806, timeout ms (25000)=1, 8:w788) -> (data out=w800:string, error out=w799:errorcluster, 3:w790:refnum<k16>)  [unwired: 1 in, 2 out]
        n293 = String Subset(string=w800, offset (0)=17 ("offset (0) 2"), length (rest)=1 ("length (rest) 2")) -> (substring=w802:string)
        n294 = String To Byte Array(string=w802) -> (unsigned byte array=w805:u8[])
        n295 = Number To Hexadecimal String(2:w805) -> (0:w804:string[])  [unwired: 1 in]
        n296 = Index Array(array=w804, index=0) -> (element=w794:string)
        n297 = Equal?(x=w794, y="F") -> (x = y?=w787:bool)
        "ROV B Enabled" <- w787
        n298 = call <vilib>:"Clear Errors.vi"("error in (no error)"=w799, "specific error code to clear (0: all)"=56) -> ("error out"=w789:errorcluster)  [unwired: 4 in, 1 out]
        n299 = Bundle By Name(cluster=w793, "connection ID"=w790, "Read ROV B"=w794) -> (w792:T5)
        n300 = call-poly <vilib>:"Select State(s)__jki_lib_state_machine.vi"("State(s) if True (\"\")"="Init: Start Timer (TMS)" ("State(s) if True (\"\")"), "Select"=w787, "State(s) if False (\"\")"="Init: Elapsed Timer (ROV B)" ("State(s) if False (\"\")")) -> ("States Out"=w791:string)  [unwired: 12 in]
        n301 = call <vilib>:"Add State(s) to Queue__jki_lib_state_machine.vi"("State(s) in Front (\"\")"=w791, "State(s) in (\"\")"=w810) -> ("States Out"=w809:string)  [unwired: 13 in]
      }
      frame "Init: Elapsed Timer (ROV B)" {
        # "check if timer elased - if TRUE end test if FALSE read again."
        # "Template Separator\n(You can make a copy of, or modify, this frame)"
        # "Check to see if the timer has elpased."
        n302 = call "Timer.vi"("error in (no error)"=w818, "Target Time"=10.0, "Enum"=T4."Get Time") -> ("error out"=w817:errorcluster, "Time Elapsed?"=w814:bool, "Elapsed Time"=→"Timeout (Read States) 2":dbl)  [unwired: 5 in, 1 out]
        n303 = call-poly <vilib>:"Select State(s)__jki_lib_state_machine.vi"("State(s) if True (\"\")"="Init: Start Timer (TMS)" ("State(s) if True (\"\")"), "Select"=w814, "State(s) if False (\"\")"="Init: Read ROV B State" ("State(s) if False (\"\")")) -> ("States Out"=w813:string)  [unwired: 12 in]
        n304 = call <vilib>:"Add State(s) to Queue__jki_lib_state_machine.vi"("State(s) in Front (\"\")"=w813, "State(s) in (\"\")"=w822) -> ("States Out"=w821:string)  [unwired: 13 in]
      }
      frame "Init: Start Timer (TMS)" {
        # "Start 10 second timer"
        # "Template Separator\n(You can make a copy of, or modify, this frame)"
        n305 = call "Timer.vi"("error in (no error)"=w829, "Enum"=T4."Start Timer") -> ("error out"=w828:errorcluster)  [unwired: 6 in, 3 out]
        n306 = property on="Timeout (Read States) 3" class="Slide (strict)"(error in=w828, "Value"=0.0 ("Horizontal Pointer Slide"), "Scale.Maximum"=10.0 ("Target Time"), "Scale.Minimum"=0.0 ("Scale.Range:Minimum")) -> (error out=w824:errorcluster)  [unwired: 1 in, 1 out]
        n307 = call <vilib>:"Add State(s) to Queue__jki_lib_state_machine.vi"("State(s) in Front (\"\")"="Init: Read TMS State" ("State(s) in Front (\"\")"), "State(s) in (\"\")"=w833) -> ("States Out"=w832:string)  [unwired: 13 in]
      }
      frame "Init: Read TMS State" {
        # "Read UDP if equal to F0 test complete if not check if timer has elapsed."
        # "#56 = didnt read before the timeout"
        # "Template Separator\n(You can make a copy of, or modify, this frame)"
        n308 = Unbundle By Name(w840) -> ("connection ID"=w853:refnum<k16>)
        n309 = UDP Read(connection ID=w853, timeout ms (25000)=1, 8:w835) -> (data out=w847:string, error out=w846:errorcluster, 3:w837:refnum<k16>)  [unwired: 1 in, 2 out]
        n310 = String Subset(string=w847, offset (0)=17 ("offset (0) 2"), length (rest)=1 ("length (rest) 2")) -> (substring=w849:string)
        n311 = String To Byte Array(string=w849) -> (unsigned byte array=w852:u8[])
        n312 = Number To Hexadecimal String(2:w852) -> (0:w851:string[])  [unwired: 1 in]
        n313 = Index Array(array=w851, index=0) -> (element=w841:string)
        n314 = Equal?(x=w841, y="12") -> (x = y?=w834:bool)
        "TMS Enabled" <- w834
        n315 = call <vilib>:"Clear Errors.vi"("error in (no error)"=w846, "specific error code to clear (0: all)"=56) -> ("error out"=w836:errorcluster)  [unwired: 4 in, 1 out]
        n316 = Bundle By Name(cluster=w840, "connection ID"=w837, "Read TMS"=w841) -> (w839:T5)
        n317 = call-poly <vilib>:"Select State(s)__jki_lib_state_machine.vi"("State(s) if True (\"\")"="Init: Start Timer (WfS)" ("State(s) if True (\"\")"), "Select"=w834, "State(s) if False (\"\")"="Init: Elapsed Timer (TMS)" ("State(s) if False (\"\")")) -> ("States Out"=w838:string)  [unwired: 12 in]
        n318 = call <vilib>:"Add State(s) to Queue__jki_lib_state_machine.vi"("State(s) in Front (\"\")"=w838, "State(s) in (\"\")"=w857) -> ("States Out"=w856:string)  [unwired: 13 in]
      }
      frame "Init: Elapsed Timer (TMS)" {
        # "check if timer elased - if TRUE end test if FALSE read again."
        # "Template Separator\n(You can make a copy of, or modify, this frame)"
        # "Check to see if the timer has elpased."
        n319 = call "Timer.vi"("error in (no error)"=w865, "Target Time"=10.0, "Enum"=T4."Get Time") -> ("error out"=w864:errorcluster, "Time Elapsed?"=w861:bool, "Elapsed Time"=→"Timeout (Read States) 3":dbl)  [unwired: 5 in, 1 out]
        n320 = call-poly <vilib>:"Select State(s)__jki_lib_state_machine.vi"("State(s) if True (\"\")"="Init: Start Timer (WfS)" ("State(s) if True (\"\")"), "Select"=w861, "State(s) if False (\"\")"="Init: Read TMS State" ("State(s) if False (\"\")")) -> ("States Out"=w860:string)  [unwired: 12 in]
        n321 = call <vilib>:"Add State(s) to Queue__jki_lib_state_machine.vi"("State(s) in Front (\"\")"=w860, "State(s) in (\"\")"=w869) -> ("States Out"=w868:string)  [unwired: 13 in]
      }
      frame "Init: Start Timer (WfS)" {
        # "Start 10 second timer"
        # "Template Separator\n(You can make a copy of, or modify, this frame)"
        n322 = call "Timer.vi"("error in (no error)"=w876, "Enum"=T4."Start Timer") -> ("error out"=w875:errorcluster)  [unwired: 6 in, 3 out]
        n323 = property on="Timeout (Read States) 4" class="Slide (strict)"(error in=w875, "Value"=0.0 ("Horizontal Pointer Slide"), "Scale.Maximum"=10.0 ("Target Time"), "Scale.Minimum"=0.0 ("Scale.Range:Minimum")) -> (error out=w871:errorcluster)  [unwired: 1 in, 1 out]
        n324 = call <vilib>:"Add State(s) to Queue__jki_lib_state_machine.vi"("State(s) in Front (\"\")"="Init: Read Wait for Start State" ("State(s) in Front (\"\")"), "State(s) in (\"\")"=w880) -> ("States Out"=w879:string)  [unwired: 13 in]
      }
      frame "Init: Read Wait for Start State" {
        # "Read UDP if equal to F0 test complete if not check if timer has elapsed."
        # "#56 = didnt read before the timeout"
        # "Template Separator\n(You can make a copy of, or modify, this frame)"
        n325 = Unbundle By Name(w887) -> ("connection ID"=w900:refnum<k16>)
        n326 = UDP Read(connection ID=w900, timeout ms (25000)=1, 8:w882) -> (data out=w894:string, error out=w893:errorcluster, 3:w884:refnum<k16>)  [unwired: 1 in, 2 out]
        n327 = String Subset(string=w894, offset (0)=17 ("offset (0) 2"), length (rest)=1 ("length (rest) 2")) -> (substring=w896:string)
        n328 = String To Byte Array(string=w896) -> (unsigned byte array=w899:u8[])
        n329 = Number To Hexadecimal String(2:w899) -> (0:w898:string[])  [unwired: 1 in]
        n330 = Index Array(array=w898, index=0) -> (element=w888:string)
        n331 = Equal?(x=w888, y="15") -> (x = y?=w881:bool)
        "Wait for Start" <- w881
        n332 = call <vilib>:"Clear Errors.vi"("error in (no error)"=w893, "specific error code to clear (0: all)"=56) -> ("error out"=w883:errorcluster)  [unwired: 4 in, 1 out]
        n333 = Bundle By Name(cluster=w887, "connection ID"=w884, "Read Wait for Start"=w888) -> (w886:T5)
        n334 = call-poly <vilib>:"Select State(s)__jki_lib_state_machine.vi"("State(s) if True (\"\")"="Init: Start Command" ("State(s) if True (\"\")"), "Select"=w881, "State(s) if False (\"\")"="Init: Elapsed Timer (WfS)" ("State(s) if False (\"\")")) -> ("States Out"=w885:string)  [unwired: 12 in]
        n335 = call <vilib>:"Add State(s) to Queue__jki_lib_state_machine.vi"("State(s) in Front (\"\")"=w885, "State(s) in (\"\")"=w904) -> ("States Out"=w903:string)  [unwired: 13 in]
      }
      frame "Init: Elapsed Timer (WfS)" {
        # "check if timer elased - if TRUE end test if FALSE read again."
        # "Template Separator\n(You can make a copy of, or modify, this frame)"
        # "Check to see if the timer has elpased."
        n336 = call "Timer.vi"("error in (no error)"=w912, "Target Time"=10.0, "Enum"=T4."Get Time") -> ("error out"=w911:errorcluster, "Time Elapsed?"=w908:bool, "Elapsed Time"=→"Timeout (Read States) 4":dbl)  [unwired: 5 in, 1 out]
        n337 = call-poly <vilib>:"Select State(s)__jki_lib_state_machine.vi"("State(s) if True (\"\")"="Init: Start Command" ("State(s) if True (\"\")"), "Select"=w908, "State(s) if False (\"\")"="Init: Read Wait for Start State" ("State(s) if False (\"\")")) -> ("States Out"=w907:string)  [unwired: 12 in]
        n338 = call <vilib>:"Add State(s) to Queue__jki_lib_state_machine.vi"("State(s) in Front (\"\")"=w907, "State(s) in (\"\")"=w916) -> ("States Out"=w915:string)  [unwired: 13 in]
      }
      frame "Init: Start Command" {
        # "None"
        # "RIB Box IP"
        # "Data"
        # "Length"
        # "ID"
        # "Target"
        # "Type"
        # "Pkt ID"
        # "SET"
        # "Template Separator\n(You can make a copy of, or modify, this frame)"
        n339 = Unbundle By Name(w935) -> ("connection ID"=w923:refnum<k16>)
        n340 = Build Array(u8 91 ("element"), u8 1 ("element"), u8 9 ("element"), u8 110 ("element"), u8 0 ("element")) -> (w933:u8[])
        n341 = Byte Array To String(unsigned byte array=w933) -> (string=w934:string)
        n342 = String To IP(1:"192.168.201.21" ("name")) -> (0:w926:u32)
        n343 = UDP Write(address=w926, port or service name=u16 54321, connection ID=w923, data in=w934, 8:w924, 9:1000 ("timeout ms (25000)")) -> (error out=w919:errorcluster, 3:w922:refnum<k16>)
        n344 = Bundle By Name(cluster=w935, "connection ID"=w922) -> (w936:T5)
        n345 = call <userlib>:"Wait (ms)__ogtk.vi"("error in (no error)"=w919, "milliseconds to wait"=u32 10000) -> ("error out"=w918:errorcluster)  [unwired: 8 in, 1 out]
        n346 = call <vilib>:"Add State(s) to Queue__jki_lib_state_machine.vi"("State(s) in Front (\"\")"="Init: Read Normal Operation" ("State(s) in Front (\"\")"), "State(s) in (\"\")"=w938) -> ("States Out"=w937:string)  [unwired: 13 in]
      }
      frame "Init: Read Normal Operation" {
        # "Read UDP if equal to F0 test complete if not check if timer has elapsed."
        # "#56 = didnt read before the timeout"
        # "Template Separator\n(You can make a copy of, or modify, this frame)"
        n347 = Unbundle By Name(w946) -> ("connection ID"=w949:refnum<k16>)
        n348 = for {
          N: 1000 -> [_]
          shift-right: [w964] -> w948
          shift-left: w945 -> [w962]
          shift-right: [w963] -> w939
          shift-left: w949 -> [w966]
          tunnel: [w954] -> w940
          stop <- w952 stop-if-true
          n349 = UDP Read(connection ID=w966, timeout ms (25000)=1, 8:w962) -> (data out=w961:string, error out=w964:errorcluster, 3:w963:refnum<k16>)  [unwired: 1 in, 2 out]
          "data out" <- w961
          n350 = String Subset(string=w961, offset (0)=17 ("offset (0) 2"), length (rest)=1 ("length (rest) 2")) -> (substring=w960:string)
          n351 = String To Byte Array(string=w960) -> (unsigned byte array=w958:u8[])
          n352 = Number To Hexadecimal String(2:w958) -> (0:w959:string[])  [unwired: 1 in]
          n353 = Index Array(array=w959, index=0) -> (element=w954:string)
          n354 = Equal?(x=w954, y="19") -> (x = y?=w952:bool)
          "Normal Operation" <- w952
        }
        n355 = Bundle By Name(cluster=w946, "connection ID"=w939, "Read Normal Operation"=w940) -> (w941:T5)
        n356 = call <vilib>:"Clear Errors.vi"("error in (no error)"=w948, "specific error code to clear (0: all)"=56) -> ("error out"=w943:errorcluster)  [unwired: 4 in, 1 out]
        n357 = call <vilib>:"Add State(s) to Queue__jki_lib_state_machine.vi"("State(s) in Front (\"\")"="Macro: Limits" ("State(s) in Front (\"\")"), "State(s) in (\"\")"=w951) -> ("States Out"=w950:string)  [unwired: 13 in]
      }
    }
    n358 = Wait (ms)(milliseconds to wait=u32 2) -> ()  [unwired: 1 out]
  }
  "error out" <- w1
